vi "JSON text to Variant.vi"(6 "LVClass Serializer":refnum<class "JSONtext LVClass Serializer.lvclass">, 8 "error in (no error)":errorcluster, 9 "Data Type":variant, 10 "Offset":i32, 11 "JSON":string) -> (0 "error out":errorcluster, 1 "Variant out":variant)   [LabVIEW 2024, in "JSONtext.lvlib"]
doc: "Convert JSON to the LabVIEW Data Type entered.\n\nStrings or Arrays of strings marked with a leading \"<JSON>\" tag in their name (including inside clusters) are returnd as JSON. \n\nStrings or Arrays of strings marked with a leading \"<UTF8>\" tag in their name (including inside clusters) are returned encoded as UTF-8 (rather than the standard LabVIEW encoding)."
uses:
  JSONtext.lvlib
  JSONtext LVClass Serializer.lvclass
  Data Type.ctl
  Unescape JSON string.vi
  Get Number Text.vi
  NaN or null to Integer ERROR.vi
  Get JSON String.vi
  Base64 or Base64URL Decode.vi
  Get String.vi
  Advance past Line Ending.vi
  Advance past Number.vi
  Advance past String.vi
  Error Cluster From Error Code.vi
  NI_Data Type.lvlib
  JDP Utility.lvlib
  SetMap.lvlib
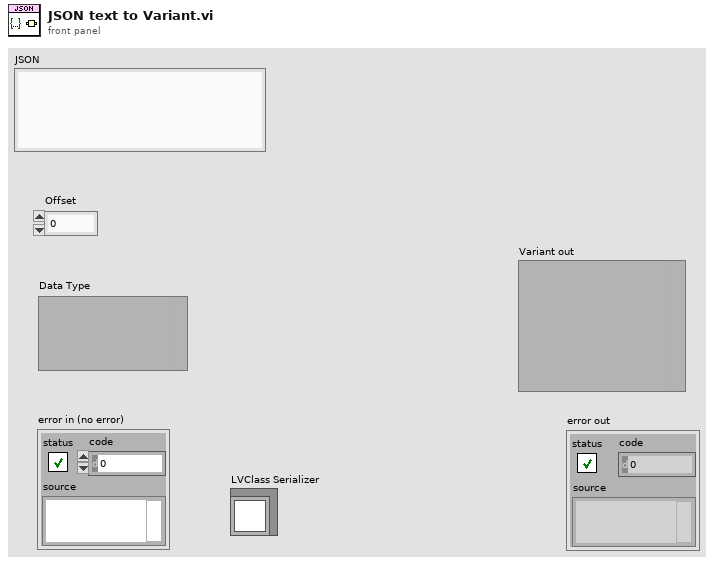
[diagram p1: front panel]
types:
  T1 = typedef "NI_Data Type.lvlib/Data Type.ctl" = enum8{"Invalid Type", "Void", "I8", "I16", "I32", "I64", "U8", "U16", "U32", "U64", "Single Float", "Double Float", "Extended Float", "Single Complex", "Double Complex", "Extended Complex", "Enum U8", "Enum U16", "Enum U32", "Enum U64", "Single Float With Unit", "Double Float With Unit", "Extended Float With Unit", "Single Complex with Unit", "Double Complex with Unit", "Extended Complex with Unit", "Boolean", "String", "Path", "Picture", "Tag", "Array", "Cluster", "Variant", "LV Variant", "Waveform", "Timestamp", "Digital Waveform", "Digital Data", "ExpressData", "Refnum", "External Data", "VI", "Poly VI", "LabVIEW Class Instance", "Fixed Point", "Set Collection", "Map Collection"}
  T2 = typedef "JSONtext.lvlib/Parsing State.ctl" = enum16{"Parser Error", "Object", "Array", "String", "Number/Other", "Leading Whitespace", "Object end", "Array end", "Value end"}
  T3 = typedef "JSONtext.lvlib/Tag Type.ctl" = enum16{"No Tag", "<JSON>", "<JOBJ>", "<UTF8>"}
  T4 = cluster{"Type":T1, "error out":errorcluster, "Tag":T3}[]
  T5 = typedef "JSONtext.lvlib/JSON Value Type.ctl" = enum16{"Not a JSON Value", "JSON Object", "JSON Array", "String", "Number", "true", "false", "null"}
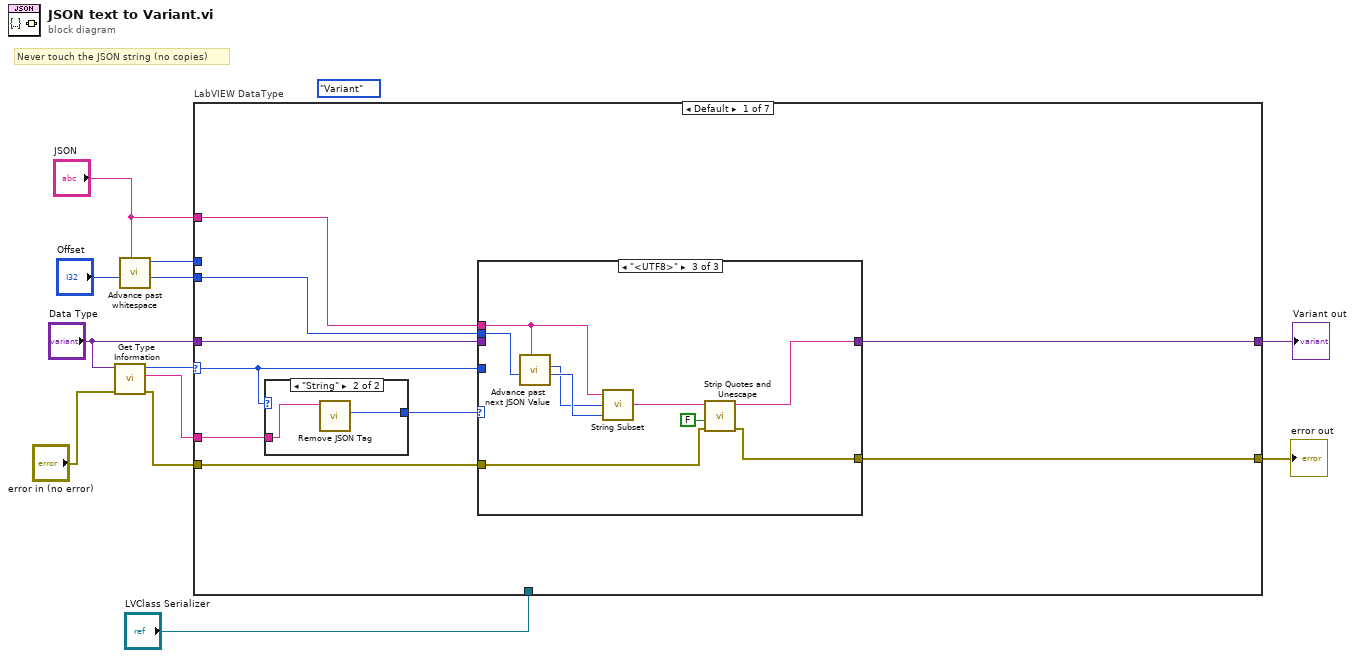
[diagram p0: block diagram]
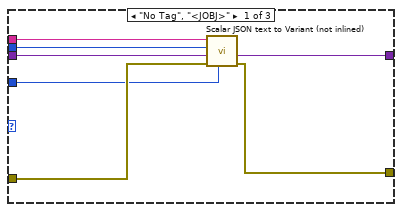
[diagram p2: hidden frame]
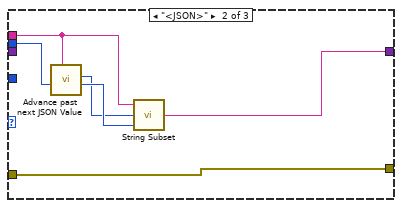
[diagram p3: hidden frame]
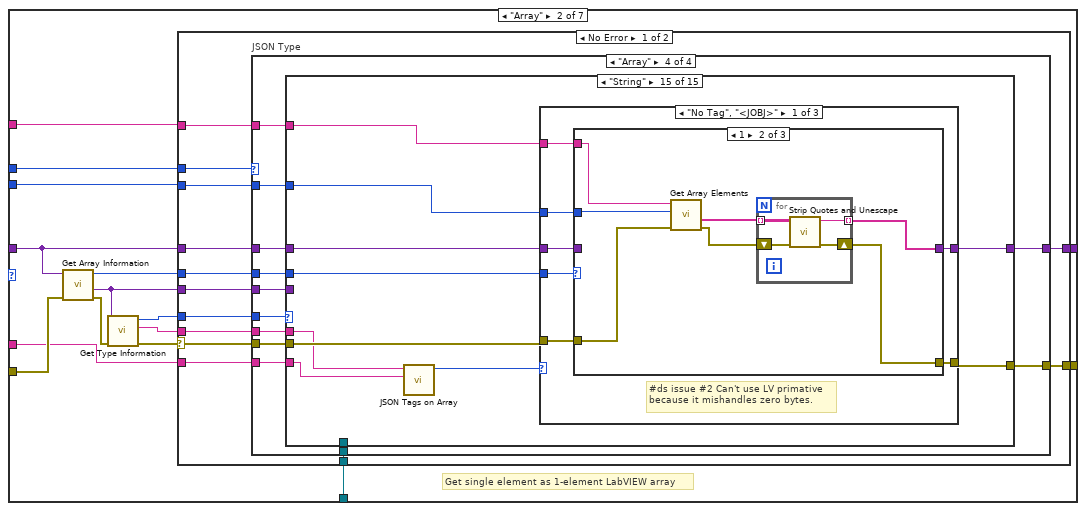
[diagram p5: hidden frame]
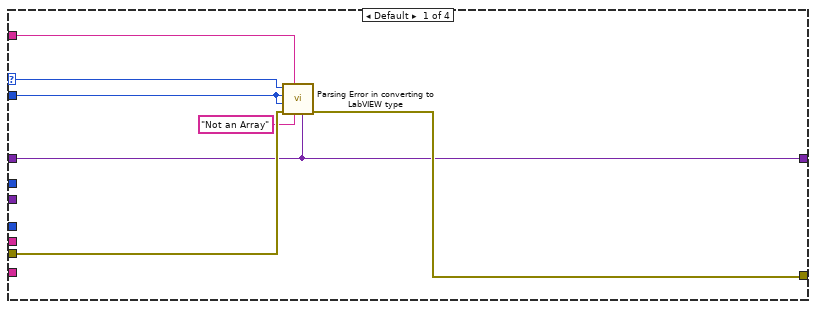
[diagram p6: hidden frame]
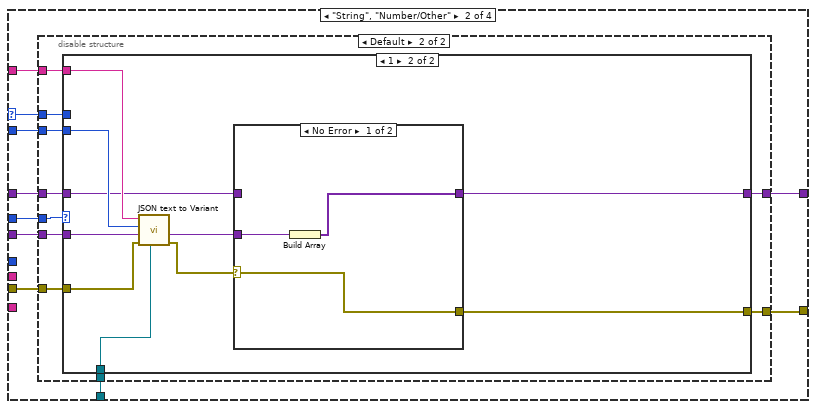
[diagram p7: hidden frame]
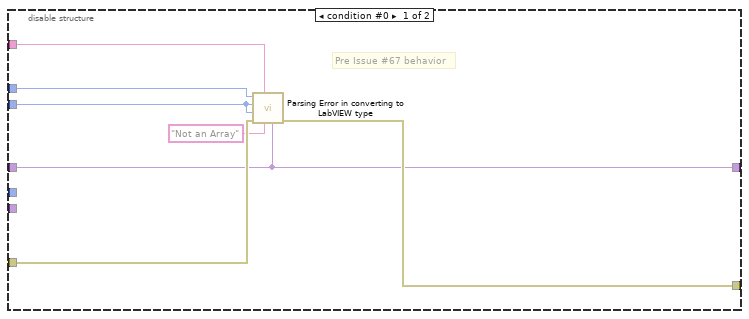
[diagram p8: hidden frame]
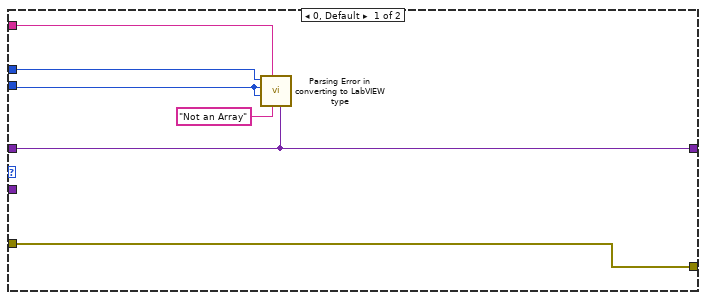
[diagram p9: hidden frame]
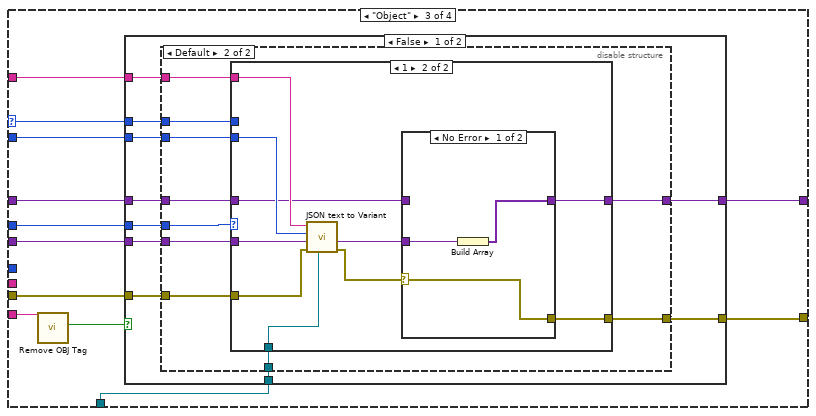
[diagram p11: hidden frame]
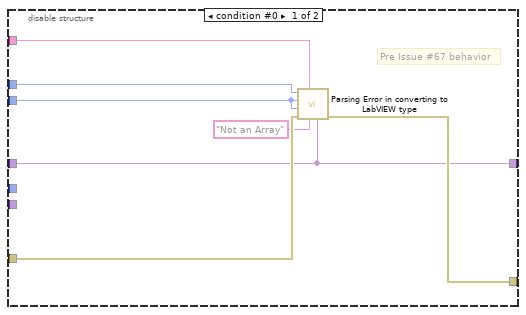
[diagram p12: hidden frame]
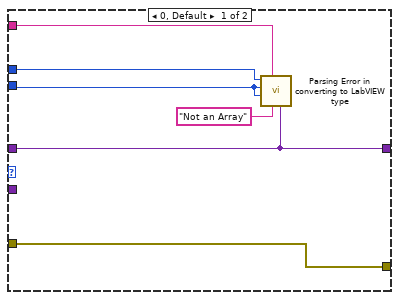
[diagram p13: hidden frame]
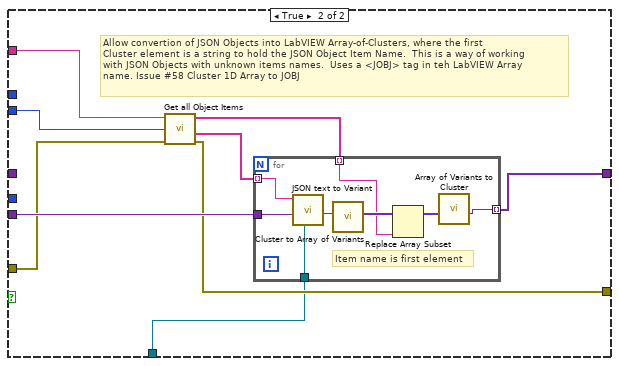
[diagram p15: hidden frame]
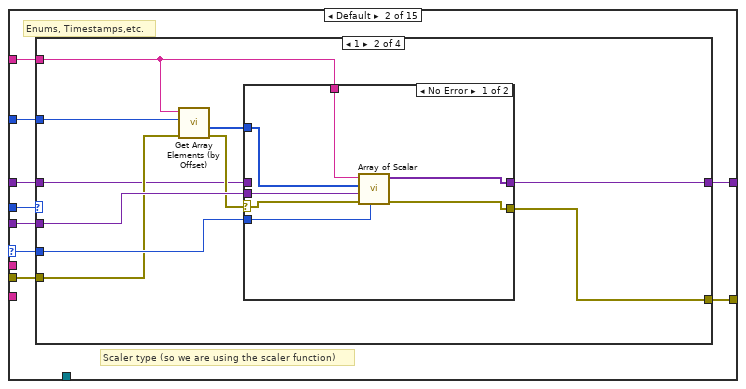
[diagram p17: hidden frame]
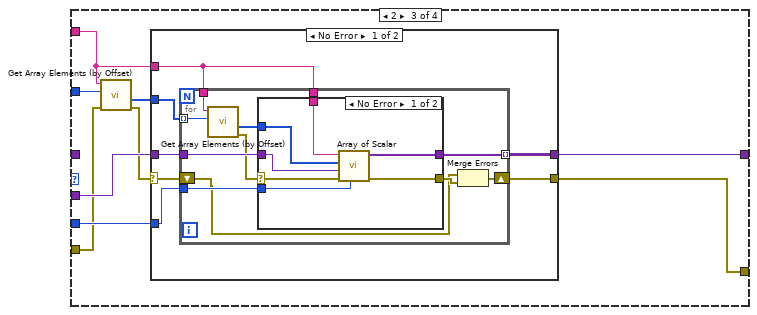
[diagram p20: hidden frame]
diagram:
  (unwired) Data_Type."Variant" ("Type")
  # "Never touch the JSON string (no copies)"
  n1 = call "Get Type Information.vi"("error in (no error)"="error in (no error)", "variant"="Data Type") -> ("error out"=w8:errorcluster, "name"=w2:string, "type"=w12:T1)  [unwired: 5 in, 2 out]
  n2 = call "Advance past whitespace.vi"("JSON"="JSON", "Offset"="Offset") -> ("Offset of first non-whitespace"=w5:i32, "Parser State"=w3:T2)  [unwired: 7 in, 1 out]
  n3 = case "LabVIEW DataType" shown="Default" w12 {
    selector: w12 -> [w14 _ _ _ _ _ w2257]
    tunnel: "Data Type" -> [w21 w53 w2187 w2195 w2226 w2237 w2259]
    tunnel: "JSON" -> [w19 w51 w2181 w2192 w2221 w2238 w2258]
    tunnel: [w16 w57 w2178 w2193 w2218 w2231 w2253] -> w9
    tunnel: w8 -> [w17 w60 w2186 w2194 w2225 w2235 w2254]
    tunnel: w5 -> [w18 w49 w2180 w2189 w2220 w2230 w2256]
    tunnel: [w20 w56 w2171 w2191 w2223 w2232 w2255] -> w7
    tunnel: w3 -> [_ w47 _ w2188 _ _ _]
    tunnel: w2 -> [w15 w50 _ _ _ _ _]
    tunnel: "LVClass Serializer" -> [_ w46 w2170 w2190 w2216 w2229 w2252]
    frame Default {
      n4 = case shown="\"String\"" w14 {
        tunnel: w15 -> [_ w45]
        tunnel: [_ w44] -> w13
        frame "Invalid Type", Default {
        }
        frame "String" {
          n5 = call "Remove JSON Tag.vi"("Name"=w45) -> ("Tag"=w44:T3)  [unwired: 9 in, 1 out]
        }
      }
      n6 = case shown="\"<UTF8>\"" w13 {
        tunnel: w21 -> [w28 _ _]
        tunnel: [w27 w30 w38] -> w20
        tunnel: w19 -> [w26 w31 w40]
        tunnel: w18 -> [w25 w34 w43]
        tunnel: w17 -> [w24 w29 w37]
        tunnel: [w23 w29 w36] -> w16
        tunnel: w14 -> [w22 _ _]
        frame "No Tag", "<JOBJ>" {
          n7 = call "Scalar JSON text to Variant (not inlined).vi"("Type"=w22, "error in (no error)"=w24, "Variant (Data Type)"=w28, "Offset (no whitespace)"=w25, "JSON"=w26) -> ("error out"=w23:errorcluster, "Variant out"=w27:variant)  [unwired: 5 in]
        }
        frame "<JSON>" {
          n8 = call "Advance past next JSON Value.vi"("JSON"=w31, "Offset"=w34) -> ("Offset out"=w33:i32, "Value start"=w32:i32)  [unwired: 7 in, 1 out]
          n9 = call "String Subset.vi"("Offset past End"=w33, "Start offset"=w32, "JSON"=w31) -> ("substring"=w30:string)  [unwired: 2 in]
        }
        frame "<UTF8>" {
          n10 = call "Advance past next JSON Value.vi"("JSON"=w40, "Offset"=w43) -> ("Offset out"=w42:i32, "Value start"=w41:i32)  [unwired: 7 in, 1 out]
          n11 = call "String Subset.vi"("Offset past End"=w42, "Start offset"=w41, "JSON"=w40) -> ("substring"=w39:string)  [unwired: 2 in]
          n12 = call "Strip Quotes and Unescape.vi"("error in (no error)"=w37, "To System Encoding (T)"=FALSE, "String"=w39) -> ("error out"=w36:errorcluster, "result string"=w38:string)  [unwired: 7 in]
        }
      }
    }
    frame "Array" {
      # "Get single element as 1-element LabVIEW array"
      n13 = call "Get Array Information.vi"("error in (no error)"=w60, "variant"=w53) -> ("error out"=w59:errorcluster, "array element data type"=w52:variant, "number of dimensions"=w54:i32)  [unwired: 6 in, 1 out]
      n14 = call "Get Type Information.vi"("error in (no error)"=w59, "variant"=w52) -> ("error out"=w58:errorcluster, "name"=w48:string, "type"=w55:T1)  [unwired: 5 in, 2 out]
      n15 = case shown="No Error" w58 {
        selector: w58 -> [w73 w2168]
        tunnel: [w72 w2168] -> w57
        tunnel: [w71 w2167] -> w56
        tunnel: w55 -> [w70 _]
        tunnel: w54 -> [w69 _]
        tunnel: w53 -> [w68 w2167]
        tunnel: w52 -> [w67 _]
        tunnel: w51 -> [w66 _]
        tunnel: w50 -> [w65 _]
        tunnel: w49 -> [w64 _]
        tunnel: w48 -> [w63 _]
        tunnel: w47 -> [w62 _]
        tunnel: w46 -> [w61 _]
        frame No Error {
          n16 = case "JSON Type" shown="\"Array\"" w62 {
            selector: w62 -> [w78 w88 w138 _]
            tunnel: w73 -> [w77 w87 w137 w217]
            tunnel: [w76 w86 w136 w216] -> w72
            tunnel: [w75 w83 w133 w215] -> w71
            tunnel: w70 -> [_ _ _ w214]
            tunnel: w69 -> [_ w82 w132 w213]
            tunnel: w68 -> [w75 w85 w135 w212]
            tunnel: w67 -> [_ w84 w134 w211]
            tunnel: w66 -> [w80 w90 w140 w210]
            tunnel: w65 -> [_ _ w130 w209]
            tunnel: w64 -> [w79 w89 w139 w208]
            tunnel: w63 -> [_ _ _ w207]
            tunnel: w61 -> [_ w81 w131 w206]
            frame Default {
              n17 = call "Parsing Error in converting to LabVIEW type.vi"("LV Type"=w75, "initial string"="Not an Array", "JSON"=w80, "error in (no error)"=w77, "Offset past match"=w79, "Value start"=w79, "State"=w78) -> ("error out"=w76:errorcluster)  [unwired: 4 in]
            }
            frame "String", "Number/Other" {
              n18 = disable-structure shown="Default" {
                disable-tunnel: w90 -> [w97 w106]
                disable-tunnel: w89 -> [w96 w105]
                disable-tunnel: w88 -> [w95 w99]
                disable-tunnel: w87 -> [w94 w104]
                disable-tunnel: [w93 w101] -> w86
                disable-tunnel: w85 -> [w91 w102]
                disable-tunnel: w84 -> [_ w107]
                disable-tunnel: [w91 w103] -> w83
                disable-tunnel: w82 -> [_ w100]
                disable-tunnel: w81 -> [_ w98]
                frame condition #0 {
                  # "Pre Issue #67 behavior"
                  n19 = call "Parsing Error in converting to LabVIEW type.vi"("LV Type"=w91, "initial string"="Not an Array", "JSON"=w97, "error in (no error)"=w94, "Offset past match"=w96, "Value start"=w96, "State"=w95) -> ("error out"=w93:errorcluster)  [unwired: 4 in]
                }
                frame condition #1 (active) {
                  n20 = case shown="1" w100 {
                    tunnel: w107 -> [_ w123]
                    tunnel: w106 -> [w112 w122]
                    tunnel: w105 -> [w110 w121]
                    tunnel: w104 -> [w108 w119]
                    tunnel: [w109 w117] -> w103
                    tunnel: w102 -> [w109 w116]
                    tunnel: [w108 w115] -> w101
                    tunnel: w99 -> [w111 _]
                    tunnel: w98 -> [_ w114]
                    frame 0, Default {
                      n21 = call "Parsing Error in converting to LabVIEW type.vi"("LV Type"=w109, "initial string"="Not an Array", "JSON"=w112, "Offset past match"=w110, "Value start"=w110, "State"=w111) -> ()  [unwired: 5 in, 1 out]
                    }
                    frame 1 {
                      n22 = call "JSON text to Variant.vi"("LVClass Serializer"=w114, "error in (no error)"=w119, "Data Type"=w123, "Offset"=w121, "JSON"=w122) -> ("error out"=w118:errorcluster, "Variant out"=w120:variant)  [unwired: 5 in]
                      n23 = case shown="No Error" w118 {
                        selector: w118 -> [w124 w127]
                        tunnel: w120 -> [w126 _]
                        tunnel: [w125 w128] -> w117
                        tunnel: w116 -> [_ w128]
                        tunnel: [w124 w127] -> w115
                        frame No Error {
                          n24 = Build Array(w126) -> (w125:variant[])
                        }
                        frame Error {
                        }
                      }
                    }
                  }
                }
              }
            }
            frame "Object" {
              n25 = call "Remove OBJ Tag.vi"("Name"=w130) -> ("tagged as Item Name in JSON Objects"=w129:bool)  [unwired: 9 in, 1 out]
              n26 = case shown="False" w129 {
                tunnel: w140 -> [w150 w195]
                tunnel: w139 -> [w149 w189]
                tunnel: w138 -> [w148 _]
                tunnel: w137 -> [w147 w196]
                tunnel: [w146 w193] -> w136
                tunnel: w135 -> [w145 _]
                tunnel: w134 -> [w144 w197]
                tunnel: [w143 w194] -> w133
                tunnel: w132 -> [w142 _]
                tunnel: w131 -> [w141 w192]
                frame False {
                  n27 = disable-structure shown="Default" {
                    disable-tunnel: w150 -> [w157 w166]
                    disable-tunnel: w149 -> [w156 w165]
                    disable-tunnel: w148 -> [w155 w159]
                    disable-tunnel: w147 -> [w154 w164]
                    disable-tunnel: [w153 w161] -> w146
                    disable-tunnel: w145 -> [w151 w162]
                    disable-tunnel: w144 -> [_ w167]
                    disable-tunnel: [w151 w163] -> w143
                    disable-tunnel: w142 -> [_ w160]
                    disable-tunnel: w141 -> [_ w158]
                    frame condition #0 {
                      # "Pre Issue #67 behavior"
                      n28 = call "Parsing Error in converting to LabVIEW type.vi"("LV Type"=w151, "initial string"="Not an Array", "JSON"=w157, "error in (no error)"=w154, "Offset past match"=w156, "Value start"=w156, "State"=w155) -> ("error out"=w153:errorcluster)  [unwired: 4 in]
                    }
                    frame condition #1 (active) {
                      n29 = case shown="1" w160 {
                        tunnel: w167 -> [_ w183]
                        tunnel: w166 -> [w172 w182]
                        tunnel: w165 -> [w170 w181]
                        tunnel: w164 -> [w168 w179]
                        tunnel: [w169 w177] -> w163
                        tunnel: w162 -> [w169 w176]
                        tunnel: [w168 w175] -> w161
                        tunnel: w159 -> [w171 _]
                        tunnel: w158 -> [_ w174]
                        frame 0, Default {
                          n30 = call "Parsing Error in converting to LabVIEW type.vi"("LV Type"=w169, "initial string"="Not an Array", "JSON"=w172, "Offset past match"=w170, "Value start"=w170, "State"=w171) -> ()  [unwired: 5 in, 1 out]
                        }
                        frame 1 {
                          n31 = call "JSON text to Variant.vi"("LVClass Serializer"=w174, "error in (no error)"=w179, "Data Type"=w183, "Offset"=w181, "JSON"=w182) -> ("error out"=w178:errorcluster, "Variant out"=w180:variant)  [unwired: 5 in]
                          n32 = case shown="No Error" w178 {
                            selector: w178 -> [w184 w187]
                            tunnel: w180 -> [w186 _]
                            tunnel: [w185 w188] -> w177
                            tunnel: w176 -> [_ w188]
                            tunnel: [w184 w187] -> w175
                            frame No Error {
                              n33 = Build Array(w186) -> (w185:variant[])
                            }
                            frame Error {
                            }
                          }
                        }
                      }
                    }
                  }
                }
                frame True {
                  # "Allow convertion of JSON Objects into LabVIEW Array-of-Clusters, where the first\nCluster element is a string to hold the JSON Object Item Name.  This is a way of working\nwith JSON Objects with unknown items names.  Uses a <JOBJ> tag in teh LabVIEW Array\nname. Issue #58 Cluster 1D Array to JOBJ"
                  n34 = call "Get all Object Items.vi"("error in (no error)"=w196, "Offset"=w189, "JSON"=w195) -> ("error out"=w193:errorcluster, "<JSON>"=w191:string[], "Item Names"=w190:string[])  [unwired: 5 in, 1 out]
                  n35 = for {
                    tunnel: w191 -> [w205] mode=indexing
                    tunnel: w197 -> [w204]
                    tunnel: w190 -> [w200] mode=indexing
                    tunnel: [w199] -> w194 mode=indexing
                    tunnel: w192 -> [w198]
                    # "Item name is first element"
                    n36 = call "JSON text to Variant.vi"("LVClass Serializer"=w198, "Data Type"=w204, "JSON"=w205) -> ("Variant out"=w202:variant)  [unwired: 7 in, 1 out]
                    n37 = call "Cluster to Array of Variants.vi"("Cluster"=w202) -> ("Array of Cluster Elements"=w201:variant[])  [unwired: 10 in]
                    n38 = Replace Array Subset(array=w201, new element=w200) -> (w203:variant[])  [unwired: 1 in]
                    n39 = call "Array of Variants to Cluster.vi"("Array of Variants"=w203) -> ("Cluster of Variants"=w199:variant)  [unwired: 10 in]
                  }
                }
              }
            }
            frame "Array" {
              n40 = case shown="\"String\"" w214 {
                selector: w214 -> [_ w220 w352 w491 w630 w769 w908 w1047 w1186 w1325 w1464 w1603 w1743 w1899 _]
                tunnel: w210 -> [_ w224 w356 w495 w634 w773 w912 w1051 w1190 w1329 w1468 w1607 w1747 w1903 w2062]
                tunnel: w217 -> [w218 w227 w359 w498 w637 w776 w915 w1054 w1193 w1332 w1471 w1610 w1750 w1906 w2061]
                tunnel: [w218 w228 w360 w499 w638 w777 w916 w1055 w1194 w1333 w1472 w1611 w1751 w1907 w2060] -> w216
                tunnel: [w219 w225 w357 w496 w635 w774 w913 w1052 w1191 w1330 w1469 w1608 w1748 w1904 w2059] -> w215
                tunnel: w213 -> [_ w223 w355 w494 w633 w772 w911 w1050 w1189 w1328 w1467 w1606 w1746 w1902 w2058]
                tunnel: w212 -> [w219 w222 w354 w493 w632 w771 w910 w1049 w1188 w1327 w1466 w1605 w1745 w1901 w2057]
                tunnel: w211 -> [_ w226 w358 w497 w636 w775 w914 w1053 w1192 w1331 w1470 w1609 w1749 w1905 _]
                tunnel: w208 -> [_ w221 w353 w492 w631 w770 w909 w1048 w1187 w1326 w1465 w1604 w1744 w1900 w2055]
                tunnel: w209 -> [_ _ _ _ _ _ _ _ _ _ _ _ _ _ w2056]
                tunnel: w207 -> [_ _ _ _ _ _ _ _ _ _ _ _ _ _ w2054]
                tunnel: w206 -> [_ _ _ _ _ _ _ _ _ _ _ _ w1742 w1898 _]
                frame "Invalid Type" {
                }
                frame Default {
                  # "Enums, Timestamps,etc."
                  # "Scaler type (so we are using the scaler function)"
                  n41 = case shown="1" w223 {
                    tunnel: [w229 w240 w254 w294] -> w228
                    tunnel: w227 -> [w229 w234 w252 w292]
                    tunnel: w226 -> [_ w239 w258 w298]
                    tunnel: [w230 w237 w256 w296] -> w225
                    tunnel: w221 -> [_ w236 w255 w295]
                    tunnel: w224 -> [_ w231 w250 w290]
                    tunnel: w222 -> [w230 w232 _ _]
                    tunnel: w220 -> [_ w235 w253 w293]
                    frame 0, Default {
                    }
                    frame 1 {
                      n42 = call "Get Array Elements (by Offset).vi"("error in (no error)"=w234, "Offset"=w236, "JSON"=w231) -> ("error out"=w233:errorcluster, "Element Offsets"=w238:i32[])  [unwired: 5 in, 2 out]
                      n43 = case shown="No Error" w233 {
                        selector: w233 -> [w243 w248]
                        tunnel: [w247 w248] -> w240
                        tunnel: w239 -> [w246 _]
                        tunnel: w238 -> [w245 _]
                        tunnel: [w244 w249] -> w237
                        tunnel: w235 -> [w241 _]
                        tunnel: w232 -> [_ w249]
                        tunnel: w231 -> [w242 _]
                        frame No Error {
                          n44 = call "Array of Scalar.vi"("Type"=w241, "error in (no error)"=w243, "Array Element Data Type"=w246, "Element Offsets"=w245, "JSON"=w242) -> ("error out"=w247:errorcluster, "Array"=w244:variant[])  [unwired: 5 in]
                        }
                        frame Error {
                        }
                      }
                    }
                    frame 2 {
                      n45 = call "Get Array Elements (by Offset).vi"("error in (no error)"=w252, "Offset"=w255, "JSON"=w250) -> ("error out"=w251:errorcluster, "Element Offsets"=w257:i32[])  [unwired: 5 in, 2 out]
                      n46 = case shown="No Error" w251 {
                        selector: w251 -> [w261 w289]
                        tunnel: w258 -> [w265 w288]
                        tunnel: w257 -> [w264 _]
                        tunnel: [w263 w288] -> w256
                        tunnel: [w259 w289] -> w254
                        tunnel: w253 -> [w262 _]
                        tunnel: w250 -> [w260 _]
                        frame No Error {
                          n47 = for {
                            tunnel: w265 -> [w275]
                            tunnel: w264 -> [w270] mode=indexing
                            tunnel: [w274] -> w263 mode=indexing
                            tunnel: w262 -> [w272]
                            tunnel: w260 -> [w269]
                            tunnel: w260 -> [w268]
                            shift-right: [w267] -> w259
                            shift-left: w261 -> [w266]
                            n48 = call "Get Array Elements (by Offset).vi"("Offset"=w270, "JSON"=w269) -> ("error out"=w271:errorcluster, "Element Offsets"=w273:i32[])  [unwired: 6 in, 2 out]
                            n49 = case shown="No Error" w271 {
                              selector: w271 -> [w279 w287]
                              tunnel: [w280 w287] -> w276
                              tunnel: w275 -> [w278 w285]
                              tunnel: [w281 w284] -> w274
                              tunnel: w273 -> [w282 _]
                              tunnel: w272 -> [w277 _]
                              tunnel: w268 -> [w283 _]
                              frame No Error {
                                n50 = call "Array of Scalar.vi"("Type"=w277, "error in (no error)"=w279, "Array Element Data Type"=w278, "Element Offsets"=w282, "JSON"=w283) -> ("error out"=w280:errorcluster, "Array"=w281:variant[])  [unwired: 5 in]
                              }
                              frame Error {
                                n51 = Initialize Array(w285, 0 ("dimension size")) -> (w284:variant[])
                              }
                            }
                            n52 = Merge Errors(w266, w276) -> (w267:errorcluster)
                          }
                        }
                        frame Error {
                        }
                      }
                    }
                    frame 3 {
                      n53 = call "Get Array Elements (by Offset).vi"("error in (no error)"=w292, "Offset"=w295, "JSON"=w290) -> ("error out"=w291:errorcluster, "Element Offsets"=w297:i32[])  [unwired: 5 in, 2 out]
                      n54 = case shown="No Error" w291 {
                        selector: w291 -> [w301 w351]
                        tunnel: w298 -> [w305 w350]
                        tunnel: w297 -> [w304 _]
                        tunnel: [w303 w350] -> w296
                        tunnel: [w299 w351] -> w294
                        tunnel: w293 -> [w302 _]
                        tunnel: w290 -> [w300 _]
                        frame No Error {
                          n55 = for {
                            tunnel: w305 -> [w315]
                            tunnel: w304 -> [w310] mode=indexing
                            tunnel: [w314] -> w303 mode=indexing
                            tunnel: w302 -> [w312]
                            tunnel: w300 -> [w309]
                            tunnel: w300 -> [w308]
                            shift-right: [w307] -> w299
                            shift-left: w301 -> [w306]
                            n56 = call "Get Array Elements (by Offset).vi"("Offset"=w310, "JSON"=w309) -> ("error out"=w311:errorcluster, "Element Offsets"=w313:i32[])  [unwired: 6 in, 2 out]
                            n57 = case shown="No Error" w311 {
                              selector: w311 -> [w317 w349]
                              tunnel: [w319 w349] -> w316
                              tunnel: w315 -> [w323 w348]
                              tunnel: [w318 w346] -> w314
                              tunnel: w313 -> [w322 _]
                              tunnel: w312 -> [w320 _]
                              tunnel: w308 -> [w321 _]
                              frame No Error {
                                n58 = for {
                                tunnel: w323 -> [w333]
                                tunnel: w322 -> [w328] mode=indexing
                                tunnel: [w332] -> w318 mode=indexing
                                tunnel: w320 -> [w330]
                                tunnel: w321 -> [w327]
                                tunnel: w321 -> [w326]
                                shift-right: [w325] -> w319
                                shift-left: w317 -> [w324]
                                n59 = call "Get Array Elements (by Offset).vi"("Offset"=w328, "JSON"=w327) -> ("error out"=w329:errorcluster, "Element Offsets"=w331:i32[])  [unwired: 6 in, 2 out]
                                n60 = case shown="No Error" w329 {
                                selector: w329 -> [w339 w345]
                                tunnel: [w340 w345] -> w334
                                tunnel: w333 -> [w338 w344]
                                tunnel: [w341 w342] -> w332
                                tunnel: w331 -> [w337 _]
                                tunnel: w330 -> [w335 _]
                                tunnel: w326 -> [w336 _]
                                frame No Error {
                                n61 = call "Array of Scalar.vi"("Type"=w335, "error in (no error)"=w339, "Array Element Data Type"=w338, "Element Offsets"=w337, "JSON"=w336) -> ("error out"=w340:errorcluster, "Array"=w341:variant[])  [unwired: 5 in]
                                }
                                frame Error {
                                n62 = Initialize Array(w344, 0 ("dimension size")) -> (w342:variant[])
                                }
                                }
                                n63 = Merge Errors(w324, w334) -> (w325:errorcluster)
                                }
                              }
                              frame Error {
                                w347 = 0 ("dimension size")
                                n64 = Initialize Array(w348, w347, w347) -> (w346:variant[][])
                              }
                            }
                            n65 = Merge Errors(w306, w316) -> (w307:errorcluster)
                          }
                        }
                        frame Error {
                        }
                      }
                    }
                  }
                }
                frame "Double Float", "Extended Float", "Double Float With Unit", "Extended Float With Unit" {
                  # "Scaler type (so we are using the inlined function)"
                  n66 = case shown="3" w355 {
                    tunnel: [w361 w372 w391 w433] -> w360
                    tunnel: w359 -> [w361 w366 w389 w431]
                    tunnel: w358 -> [_ w371 w395 w437]
                    tunnel: [w362 w369 w393 w435] -> w357
                    tunnel: w353 -> [_ w368 w392 w434]
                    tunnel: w356 -> [_ w363 w387 w429]
                    tunnel: w354 -> [w362 w364 _ _]
                    tunnel: w352 -> [_ w367 w390 w432]
                    frame 0, Default {
                    }
                    frame 1 {
                      n67 = call "Get Array Elements (by Offset).vi"("error in (no error)"=w366, "Offset"=w368, "JSON"=w363) -> ("error out"=w365:errorcluster, "Element Offsets"=w370:i32[])  [unwired: 5 in, 2 out]
                      n68 = case shown="No Error" w365 {
                        selector: w365 -> [w374 w386]
                        tunnel: [w379 w386] -> w372
                        tunnel: w371 -> [w378 _]
                        tunnel: w370 -> [w377 _]
                        tunnel: [w376 _] -> w369
                        tunnel: w367 -> [w375 _]
                        tunnel: w364 -> [_ _]
                        tunnel: w363 -> [w373 _]
                        frame No Error {
                          n69 = for {
                            tunnel: w378 -> [_]
                            tunnel: [w381] -> w376 mode=indexing
                            tunnel: w377 -> [w382] mode=indexing
                            tunnel: w375 -> [_]
                            tunnel: w373 -> [w383]
                            shift-right: [w385] -> w379
                            shift-left: w374 -> [w384]
                            n70 = call "Get DBL.vi"("Offset"=w382, "JSON"=w383) -> ("error out"=w380:errorcluster, "Number"=w381:dbl)  [unwired: 7 in, 1 out]
                            n71 = Merge Errors(w384, w380) -> (w385:errorcluster)
                          }
                        }
                        frame Error {
                        }
                      }
                    }
                    frame 2 {
                      n72 = call "Get Array Elements (by Offset).vi"("error in (no error)"=w389, "Offset"=w392, "JSON"=w387) -> ("error out"=w388:errorcluster, "Element Offsets"=w394:i32[])  [unwired: 5 in, 2 out]
                      n73 = case shown="No Error" w388 {
                        selector: w388 -> [w398 w428]
                        tunnel: w395 -> [w402 _]
                        tunnel: w394 -> [w401 _]
                        tunnel: [w400 _] -> w393
                        tunnel: [w396 w428] -> w391
                        tunnel: w390 -> [w399 _]
                        tunnel: w387 -> [w397 _]
                        frame No Error {
                          n74 = for {
                            tunnel: w402 -> [w412]
                            tunnel: w401 -> [w407] mode=indexing
                            tunnel: [w411] -> w400 mode=indexing
                            tunnel: w399 -> [w409]
                            tunnel: w397 -> [w406]
                            tunnel: w397 -> [w405]
                            shift-right: [w404] -> w396
                            shift-left: w398 -> [w403]
                            n75 = call "Get Array Elements (by Offset).vi"("Offset"=w407, "JSON"=w406) -> ("error out"=w408:errorcluster, "Element Offsets"=w410:i32[])  [unwired: 6 in, 2 out]
                            n76 = case shown="No Error" w408 {
                              selector: w408 -> [w416 w427]
                              tunnel: [w414 w427] -> w413
                              tunnel: w412 -> [w420 _]
                              tunnel: [w419 _] -> w411
                              tunnel: w410 -> [w418 _]
                              tunnel: w409 -> [w417 _]
                              tunnel: w405 -> [w415 _]
                              frame No Error {
                                n77 = for {
                                tunnel: w420 -> [_]
                                tunnel: [w421] -> w419 mode=indexing
                                tunnel: w418 -> [w423] mode=indexing
                                tunnel: w417 -> [_]
                                tunnel: w415 -> [w424]
                                shift-right: [w426] -> w414
                                shift-left: w416 -> [w425]
                                n78 = call "Get DBL.vi"("Offset"=w423, "JSON"=w424) -> ("error out"=w422:errorcluster, "Number"=w421:dbl)  [unwired: 7 in, 1 out]
                                n79 = Merge Errors(w425, w422) -> (w426:errorcluster)
                                }
                              }
                              frame Error {
                              }
                            }
                            n80 = Merge Errors(w403, w413) -> (w404:errorcluster)
                          }
                        }
                        frame Error {
                        }
                      }
                    }
                    frame 3 {
                      n81 = call "Get Array Elements (by Offset).vi"("error in (no error)"=w431, "Offset"=w434, "JSON"=w429) -> ("error out"=w430:errorcluster, "Element Offsets"=w436:i32[])  [unwired: 5 in, 2 out]
                      n82 = case shown="No Error" w430 {
                        selector: w430 -> [w440 w490]
                        tunnel: w437 -> [w444 w489]
                        tunnel: w436 -> [w443 _]
                        tunnel: [w442 w489] -> w435
                        tunnel: [w438 w490] -> w433
                        tunnel: w432 -> [w441 _]
                        tunnel: w429 -> [w439 _]
                        frame No Error {
                          n83 = for {
                            tunnel: w444 -> [w454]
                            tunnel: w443 -> [w449] mode=indexing
                            tunnel: [w453] -> w442 mode=indexing
                            tunnel: w441 -> [w451]
                            tunnel: w439 -> [w448]
                            tunnel: w439 -> [w447]
                            shift-right: [w446] -> w438
                            shift-left: w440 -> [w445]
                            n84 = call "Get Array Elements (by Offset).vi"("Offset"=w449, "JSON"=w448) -> ("error out"=w450:errorcluster, "Element Offsets"=w452:i32[])  [unwired: 6 in, 2 out]
                            n85 = case shown="No Error" w450 {
                              selector: w450 -> [w456 w488]
                              tunnel: [w458 w488] -> w455
                              tunnel: w454 -> [w462 _]
                              tunnel: [w457 _] -> w453
                              tunnel: w452 -> [w461 _]
                              tunnel: w451 -> [w459 _]
                              tunnel: w447 -> [w460 _]
                              frame No Error {
                                n86 = for {
                                tunnel: w462 -> [w472]
                                tunnel: w461 -> [w467] mode=indexing
                                tunnel: [w471] -> w457 mode=indexing
                                tunnel: w459 -> [w469]
                                tunnel: w460 -> [w466]
                                tunnel: w460 -> [w465]
                                shift-right: [w464] -> w458
                                shift-left: w456 -> [w463]
                                n87 = call "Get Array Elements (by Offset).vi"("Offset"=w467, "JSON"=w466) -> ("error out"=w468:errorcluster, "Element Offsets"=w470:i32[])  [unwired: 6 in, 2 out]
                                n88 = case shown="No Error" w468 {
                                selector: w468 -> [w476 w487]
                                tunnel: [w474 w487] -> w473
                                tunnel: w472 -> [w480 _]
                                tunnel: [w479 _] -> w471
                                tunnel: w470 -> [w478 _]
                                tunnel: w469 -> [w477 _]
                                tunnel: w465 -> [w475 _]
                                frame No Error {
                                n89 = for {
                                tunnel: w480 -> [_]
                                tunnel: [w481] -> w479 mode=indexing
                                tunnel: w478 -> [w484] mode=indexing
                                tunnel: w477 -> [_]
                                tunnel: w475 -> [w485]
                                shift-right: [w486] -> w474
                                shift-left: w476 -> [w483]
                                n90 = call "Get DBL.vi"("Offset"=w484, "JSON"=w485) -> ("error out"=w482:errorcluster, "Number"=w481:dbl)  [unwired: 7 in, 1 out]
                                n91 = Merge Errors(w483, w482) -> (w486:errorcluster)
                                }
                                }
                                frame Error {
                                }
                                }
                                n92 = Merge Errors(w463, w473) -> (w464:errorcluster)
                                }
                              }
                              frame Error {
                              }
                            }
                            n93 = Merge Errors(w445, w455) -> (w446:errorcluster)
                          }
                        }
                        frame Error {
                        }
                      }
                    }
                  }
                }
                frame "Single Float", "Single Float With Unit" {
                  # "Scaler type (so we are using the inlined function)"
                  n94 = case shown="3" w494 {
                    tunnel: [w500 w511 w530 w572] -> w499
                    tunnel: w498 -> [w500 w505 w528 w570]
                    tunnel: w497 -> [_ w510 w534 w576]
                    tunnel: [w501 w508 w532 w574] -> w496
                    tunnel: w492 -> [_ w507 w531 w573]
                    tunnel: w495 -> [_ w502 w526 w568]
                    tunnel: w493 -> [w501 w503 _ _]
                    tunnel: w491 -> [_ w506 w529 w571]
                    frame 0, Default {
                    }
                    frame 1 {
                      n95 = call "Get Array Elements (by Offset).vi"("error in (no error)"=w505, "Offset"=w507, "JSON"=w502) -> ("error out"=w504:errorcluster, "Element Offsets"=w509:i32[])  [unwired: 5 in, 2 out]
                      n96 = case shown="No Error" w504 {
                        selector: w504 -> [w513 w525]
                        tunnel: [w518 w525] -> w511
                        tunnel: w510 -> [w517 _]
                        tunnel: w509 -> [w516 _]
                        tunnel: [w515 _] -> w508
                        tunnel: w506 -> [w514 _]
                        tunnel: w503 -> [_ _]
                        tunnel: w502 -> [w512 _]
                        frame No Error {
                          n97 = for {
                            tunnel: w517 -> [_]
                            tunnel: [w520] -> w515 mode=indexing
                            tunnel: w516 -> [w521] mode=indexing
                            tunnel: w514 -> [_]
                            tunnel: w512 -> [w522]
                            shift-right: [w524] -> w518
                            shift-left: w513 -> [w523]
                            n98 = call "Get SGL.vi"("Offset"=w521, "JSON"=w522) -> ("error out"=w519:errorcluster, "Number"=w520:sgl)  [unwired: 7 in, 1 out]
                            n99 = Merge Errors(w523, w519) -> (w524:errorcluster)
                          }
                        }
                        frame Error {
                        }
                      }
                    }
                    frame 2 {
                      n100 = call "Get Array Elements (by Offset).vi"("error in (no error)"=w528, "Offset"=w531, "JSON"=w526) -> ("error out"=w527:errorcluster, "Element Offsets"=w533:i32[])  [unwired: 5 in, 2 out]
                      n101 = case shown="No Error" w527 {
                        selector: w527 -> [w537 w567]
                        tunnel: w534 -> [w541 _]
                        tunnel: w533 -> [w540 _]
                        tunnel: [w539 _] -> w532
                        tunnel: [w535 w567] -> w530
                        tunnel: w529 -> [w538 _]
                        tunnel: w526 -> [w536 _]
                        frame No Error {
                          n102 = for {
                            tunnel: w541 -> [w551]
                            tunnel: w540 -> [w546] mode=indexing
                            tunnel: [w550] -> w539 mode=indexing
                            tunnel: w538 -> [w548]
                            tunnel: w536 -> [w545]
                            tunnel: w536 -> [w544]
                            shift-right: [w543] -> w535
                            shift-left: w537 -> [w542]
                            n103 = call "Get Array Elements (by Offset).vi"("Offset"=w546, "JSON"=w545) -> ("error out"=w547:errorcluster, "Element Offsets"=w549:i32[])  [unwired: 6 in, 2 out]
                            n104 = case shown="No Error" w547 {
                              selector: w547 -> [w555 w566]
                              tunnel: [w553 w566] -> w552
                              tunnel: w551 -> [w559 _]
                              tunnel: [w558 _] -> w550
                              tunnel: w549 -> [w557 _]
                              tunnel: w548 -> [w556 _]
                              tunnel: w544 -> [w554 _]
                              frame No Error {
                                n105 = for {
                                tunnel: w559 -> [_]
                                tunnel: [w560] -> w558 mode=indexing
                                tunnel: w557 -> [w562] mode=indexing
                                tunnel: w556 -> [_]
                                tunnel: w554 -> [w563]
                                shift-right: [w565] -> w553
                                shift-left: w555 -> [w564]
                                n106 = call "Get SGL.vi"("Offset"=w562, "JSON"=w563) -> ("error out"=w561:errorcluster, "Number"=w560:sgl)  [unwired: 7 in, 1 out]
                                n107 = Merge Errors(w564, w561) -> (w565:errorcluster)
                                }
                              }
                              frame Error {
                              }
                            }
                            n108 = Merge Errors(w542, w552) -> (w543:errorcluster)
                          }
                        }
                        frame Error {
                        }
                      }
                    }
                    frame 3 {
                      n109 = call "Get Array Elements (by Offset).vi"("error in (no error)"=w570, "Offset"=w573, "JSON"=w568) -> ("error out"=w569:errorcluster, "Element Offsets"=w575:i32[])  [unwired: 5 in, 2 out]
                      n110 = case shown="No Error" w569 {
                        selector: w569 -> [w579 w629]
                        tunnel: w576 -> [w583 w628]
                        tunnel: w575 -> [w582 _]
                        tunnel: [w581 w628] -> w574
                        tunnel: [w577 w629] -> w572
                        tunnel: w571 -> [w580 _]
                        tunnel: w568 -> [w578 _]
                        frame No Error {
                          n111 = for {
                            tunnel: w583 -> [w593]
                            tunnel: w582 -> [w588] mode=indexing
                            tunnel: [w592] -> w581 mode=indexing
                            tunnel: w580 -> [w590]
                            tunnel: w578 -> [w587]
                            tunnel: w578 -> [w586]
                            shift-right: [w585] -> w577
                            shift-left: w579 -> [w584]
                            n112 = call "Get Array Elements (by Offset).vi"("Offset"=w588, "JSON"=w587) -> ("error out"=w589:errorcluster, "Element Offsets"=w591:i32[])  [unwired: 6 in, 2 out]
                            n113 = case shown="No Error" w589 {
                              selector: w589 -> [w595 w627]
                              tunnel: [w597 w627] -> w594
                              tunnel: w593 -> [w601 _]
                              tunnel: [w596 _] -> w592
                              tunnel: w591 -> [w600 _]
                              tunnel: w590 -> [w598 _]
                              tunnel: w586 -> [w599 _]
                              frame No Error {
                                n114 = for {
                                tunnel: w601 -> [w611]
                                tunnel: w600 -> [w606] mode=indexing
                                tunnel: [w610] -> w596 mode=indexing
                                tunnel: w598 -> [w608]
                                tunnel: w599 -> [w605]
                                tunnel: w599 -> [w604]
                                shift-right: [w603] -> w597
                                shift-left: w595 -> [w602]
                                n115 = call "Get Array Elements (by Offset).vi"("Offset"=w606, "JSON"=w605) -> ("error out"=w607:errorcluster, "Element Offsets"=w609:i32[])  [unwired: 6 in, 2 out]
                                n116 = case shown="No Error" w607 {
                                selector: w607 -> [w615 w626]
                                tunnel: [w613 w626] -> w612
                                tunnel: w611 -> [w619 _]
                                tunnel: [w618 _] -> w610
                                tunnel: w609 -> [w617 _]
                                tunnel: w608 -> [w616 _]
                                tunnel: w604 -> [w614 _]
                                frame No Error {
                                n117 = for {
                                tunnel: w619 -> [_]
                                tunnel: [w620] -> w618 mode=indexing
                                tunnel: w617 -> [w623] mode=indexing
                                tunnel: w616 -> [_]
                                tunnel: w614 -> [w624]
                                shift-right: [w625] -> w613
                                shift-left: w615 -> [w622]
                                n118 = call "Get SGL.vi"("Offset"=w623, "JSON"=w624) -> ("error out"=w621:errorcluster, "Number"=w620:sgl)  [unwired: 7 in, 1 out]
                                n119 = Merge Errors(w622, w621) -> (w625:errorcluster)
                                }
                                }
                                frame Error {
                                }
                                }
                                n120 = Merge Errors(w602, w612) -> (w603:errorcluster)
                                }
                              }
                              frame Error {
                              }
                            }
                            n121 = Merge Errors(w584, w594) -> (w585:errorcluster)
                          }
                        }
                        frame Error {
                        }
                      }
                    }
                  }
                }
                frame "I8" {
                  n122 = case shown="3" w633 {
                    tunnel: [w639 w650 w669 w711] -> w638
                    tunnel: w637 -> [w639 w644 w667 w709]
                    tunnel: w636 -> [_ w649 w673 w715]
                    tunnel: [w640 w647 w671 w713] -> w635
                    tunnel: w631 -> [_ w646 w670 w712]
                    tunnel: w634 -> [_ w641 w665 w707]
                    tunnel: w632 -> [w640 w642 _ _]
                    tunnel: w630 -> [_ w645 w668 w710]
                    frame 0, Default {
                    }
                    frame 1 {
                      n123 = call "Get Array Elements (by Offset).vi"("error in (no error)"=w644, "Offset"=w646, "JSON"=w641) -> ("error out"=w643:errorcluster, "Element Offsets"=w648:i32[])  [unwired: 5 in, 2 out]
                      n124 = case shown="No Error" w643 {
                        selector: w643 -> [w652 w664]
                        tunnel: [w657 w664] -> w650
                        tunnel: w649 -> [w656 _]
                        tunnel: w648 -> [w655 _]
                        tunnel: [w654 _] -> w647
                        tunnel: w645 -> [w653 _]
                        tunnel: w642 -> [_ _]
                        tunnel: w641 -> [w651 _]
                        frame No Error {
                          n125 = for {
                            tunnel: w656 -> [_]
                            tunnel: [w659] -> w654 mode=indexing
                            tunnel: w655 -> [w660] mode=indexing
                            tunnel: w653 -> [_]
                            tunnel: w651 -> [w661]
                            shift-right: [w663] -> w657
                            shift-left: w652 -> [w662]
                            n126 = call "Get I8.vi"("Offset"=w660, "JSON"=w661) -> ("error out"=w658:errorcluster, "Number"=w659:i8)  [unwired: 7 in, 1 out]
                            n127 = Merge Errors(w662, w658) -> (w663:errorcluster)
                          }
                        }
                        frame Error {
                        }
                      }
                    }
                    frame 2 {
                      n128 = call "Get Array Elements (by Offset).vi"("error in (no error)"=w667, "Offset"=w670, "JSON"=w665) -> ("error out"=w666:errorcluster, "Element Offsets"=w672:i32[])  [unwired: 5 in, 2 out]
                      n129 = case shown="No Error" w666 {
                        selector: w666 -> [w676 w706]
                        tunnel: w673 -> [w680 _]
                        tunnel: w672 -> [w679 _]
                        tunnel: [w678 _] -> w671
                        tunnel: [w674 w706] -> w669
                        tunnel: w668 -> [w677 _]
                        tunnel: w665 -> [w675 _]
                        frame No Error {
                          n130 = for {
                            tunnel: w680 -> [w690]
                            tunnel: w679 -> [w685] mode=indexing
                            tunnel: [w689] -> w678 mode=indexing
                            tunnel: w677 -> [w687]
                            tunnel: w675 -> [w684]
                            tunnel: w675 -> [w683]
                            shift-right: [w682] -> w674
                            shift-left: w676 -> [w681]
                            n131 = call "Get Array Elements (by Offset).vi"("Offset"=w685, "JSON"=w684) -> ("error out"=w686:errorcluster, "Element Offsets"=w688:i32[])  [unwired: 6 in, 2 out]
                            n132 = case shown="No Error" w686 {
                              selector: w686 -> [w694 w705]
                              tunnel: [w692 w705] -> w691
                              tunnel: w690 -> [w698 _]
                              tunnel: [w697 _] -> w689
                              tunnel: w688 -> [w696 _]
                              tunnel: w687 -> [w695 _]
                              tunnel: w683 -> [w693 _]
                              frame No Error {
                                n133 = for {
                                tunnel: w698 -> [_]
                                tunnel: [w699] -> w697 mode=indexing
                                tunnel: w696 -> [w701] mode=indexing
                                tunnel: w695 -> [_]
                                tunnel: w693 -> [w702]
                                shift-right: [w704] -> w692
                                shift-left: w694 -> [w703]
                                n134 = call "Get I8.vi"("Offset"=w701, "JSON"=w702) -> ("error out"=w700:errorcluster, "Number"=w699:i8)  [unwired: 7 in, 1 out]
                                n135 = Merge Errors(w703, w700) -> (w704:errorcluster)
                                }
                              }
                              frame Error {
                              }
                            }
                            n136 = Merge Errors(w681, w691) -> (w682:errorcluster)
                          }
                        }
                        frame Error {
                        }
                      }
                    }
                    frame 3 {
                      n137 = call "Get Array Elements (by Offset).vi"("error in (no error)"=w709, "Offset"=w712, "JSON"=w707) -> ("error out"=w708:errorcluster, "Element Offsets"=w714:i32[])  [unwired: 5 in, 2 out]
                      n138 = case shown="No Error" w708 {
                        selector: w708 -> [w718 w768]
                        tunnel: w715 -> [w722 w767]
                        tunnel: w714 -> [w721 _]
                        tunnel: [w720 w767] -> w713
                        tunnel: [w716 w768] -> w711
                        tunnel: w710 -> [w719 _]
                        tunnel: w707 -> [w717 _]
                        frame No Error {
                          n139 = for {
                            tunnel: w722 -> [w732]
                            tunnel: w721 -> [w727] mode=indexing
                            tunnel: [w731] -> w720 mode=indexing
                            tunnel: w719 -> [w729]
                            tunnel: w717 -> [w726]
                            tunnel: w717 -> [w725]
                            shift-right: [w724] -> w716
                            shift-left: w718 -> [w723]
                            n140 = call "Get Array Elements (by Offset).vi"("Offset"=w727, "JSON"=w726) -> ("error out"=w728:errorcluster, "Element Offsets"=w730:i32[])  [unwired: 6 in, 2 out]
                            n141 = case shown="No Error" w728 {
                              selector: w728 -> [w734 w766]
                              tunnel: [w736 w766] -> w733
                              tunnel: w732 -> [w740 _]
                              tunnel: [w735 _] -> w731
                              tunnel: w730 -> [w739 _]
                              tunnel: w729 -> [w737 _]
                              tunnel: w725 -> [w738 _]
                              frame No Error {
                                n142 = for {
                                tunnel: w740 -> [w750]
                                tunnel: w739 -> [w745] mode=indexing
                                tunnel: [w749] -> w735 mode=indexing
                                tunnel: w737 -> [w747]
                                tunnel: w738 -> [w744]
                                tunnel: w738 -> [w743]
                                shift-right: [w742] -> w736
                                shift-left: w734 -> [w741]
                                n143 = call "Get Array Elements (by Offset).vi"("Offset"=w745, "JSON"=w744) -> ("error out"=w746:errorcluster, "Element Offsets"=w748:i32[])  [unwired: 6 in, 2 out]
                                n144 = case shown="No Error" w746 {
                                selector: w746 -> [w754 w765]
                                tunnel: [w752 w765] -> w751
                                tunnel: w750 -> [w758 _]
                                tunnel: [w757 _] -> w749
                                tunnel: w748 -> [w756 _]
                                tunnel: w747 -> [w755 _]
                                tunnel: w743 -> [w753 _]
                                frame No Error {
                                n145 = for {
                                tunnel: w758 -> [_]
                                tunnel: [w759] -> w757 mode=indexing
                                tunnel: w756 -> [w762] mode=indexing
                                tunnel: w755 -> [_]
                                tunnel: w753 -> [w763]
                                shift-right: [w764] -> w752
                                shift-left: w754 -> [w761]
                                n146 = call "Get I8.vi"("Offset"=w762, "JSON"=w763) -> ("error out"=w760:errorcluster, "Number"=w759:i8)  [unwired: 7 in, 1 out]
                                n147 = Merge Errors(w761, w760) -> (w764:errorcluster)
                                }
                                }
                                frame Error {
                                }
                                }
                                n148 = Merge Errors(w741, w751) -> (w742:errorcluster)
                                }
                              }
                              frame Error {
                              }
                            }
                            n149 = Merge Errors(w723, w733) -> (w724:errorcluster)
                          }
                        }
                        frame Error {
                        }
                      }
                    }
                  }
                }
                frame "I16" {
                  # "Scaler type (so we are using the inlined function)"
                  n150 = case shown="3" w772 {
                    tunnel: [w778 w789 w808 w850] -> w777
                    tunnel: w776 -> [w778 w783 w806 w848]
                    tunnel: w775 -> [_ w788 w812 w854]
                    tunnel: [w779 w786 w810 w852] -> w774
                    tunnel: w770 -> [_ w785 w809 w851]
                    tunnel: w773 -> [_ w780 w804 w846]
                    tunnel: w771 -> [w779 w781 _ _]
                    tunnel: w769 -> [_ w784 w807 w849]
                    frame 0, Default {
                    }
                    frame 1 {
                      n151 = call "Get Array Elements (by Offset).vi"("error in (no error)"=w783, "Offset"=w785, "JSON"=w780) -> ("error out"=w782:errorcluster, "Element Offsets"=w787:i32[])  [unwired: 5 in, 2 out]
                      n152 = case shown="No Error" w782 {
                        selector: w782 -> [w791 w803]
                        tunnel: [w796 w803] -> w789
                        tunnel: w788 -> [w795 _]
                        tunnel: w787 -> [w794 _]
                        tunnel: [w793 _] -> w786
                        tunnel: w784 -> [w792 _]
                        tunnel: w781 -> [_ _]
                        tunnel: w780 -> [w790 _]
                        frame No Error {
                          n153 = for {
                            tunnel: w795 -> [_]
                            tunnel: [w798] -> w793 mode=indexing
                            tunnel: w794 -> [w799] mode=indexing
                            tunnel: w792 -> [_]
                            tunnel: w790 -> [w800]
                            shift-right: [w802] -> w796
                            shift-left: w791 -> [w801]
                            n154 = call "Get I16.vi"("Offset"=w799, "JSON"=w800) -> ("error out"=w797:errorcluster, "Number"=w798:i16)  [unwired: 7 in, 1 out]
                            n155 = Merge Errors(w801, w797) -> (w802:errorcluster)
                          }
                        }
                        frame Error {
                        }
                      }
                    }
                    frame 2 {
                      n156 = call "Get Array Elements (by Offset).vi"("error in (no error)"=w806, "Offset"=w809, "JSON"=w804) -> ("error out"=w805:errorcluster, "Element Offsets"=w811:i32[])  [unwired: 5 in, 2 out]
                      n157 = case shown="No Error" w805 {
                        selector: w805 -> [w815 w845]
                        tunnel: w812 -> [w819 _]
                        tunnel: w811 -> [w818 _]
                        tunnel: [w817 _] -> w810
                        tunnel: [w813 w845] -> w808
                        tunnel: w807 -> [w816 _]
                        tunnel: w804 -> [w814 _]
                        frame No Error {
                          n158 = for {
                            tunnel: w819 -> [w829]
                            tunnel: w818 -> [w824] mode=indexing
                            tunnel: [w828] -> w817 mode=indexing
                            tunnel: w816 -> [w826]
                            tunnel: w814 -> [w823]
                            tunnel: w814 -> [w822]
                            shift-right: [w821] -> w813
                            shift-left: w815 -> [w820]
                            n159 = call "Get Array Elements (by Offset).vi"("Offset"=w824, "JSON"=w823) -> ("error out"=w825:errorcluster, "Element Offsets"=w827:i32[])  [unwired: 6 in, 2 out]
                            n160 = case shown="No Error" w825 {
                              selector: w825 -> [w833 w844]
                              tunnel: [w831 w844] -> w830
                              tunnel: w829 -> [w837 _]
                              tunnel: [w836 _] -> w828
                              tunnel: w827 -> [w835 _]
                              tunnel: w826 -> [w834 _]
                              tunnel: w822 -> [w832 _]
                              frame No Error {
                                n161 = for {
                                tunnel: w837 -> [_]
                                tunnel: [w838] -> w836 mode=indexing
                                tunnel: w835 -> [w840] mode=indexing
                                tunnel: w834 -> [_]
                                tunnel: w832 -> [w841]
                                shift-right: [w843] -> w831
                                shift-left: w833 -> [w842]
                                n162 = call "Get I16.vi"("Offset"=w840, "JSON"=w841) -> ("error out"=w839:errorcluster, "Number"=w838:i16)  [unwired: 7 in, 1 out]
                                n163 = Merge Errors(w842, w839) -> (w843:errorcluster)
                                }
                              }
                              frame Error {
                              }
                            }
                            n164 = Merge Errors(w820, w830) -> (w821:errorcluster)
                          }
                        }
                        frame Error {
                        }
                      }
                    }
                    frame 3 {
                      n165 = call "Get Array Elements (by Offset).vi"("error in (no error)"=w848, "Offset"=w851, "JSON"=w846) -> ("error out"=w847:errorcluster, "Element Offsets"=w853:i32[])  [unwired: 5 in, 2 out]
                      n166 = case shown="No Error" w847 {
                        selector: w847 -> [w857 w907]
                        tunnel: w854 -> [w861 w906]
                        tunnel: w853 -> [w860 _]
                        tunnel: [w859 w906] -> w852
                        tunnel: [w855 w907] -> w850
                        tunnel: w849 -> [w858 _]
                        tunnel: w846 -> [w856 _]
                        frame No Error {
                          n167 = for {
                            tunnel: w861 -> [w871]
                            tunnel: w860 -> [w866] mode=indexing
                            tunnel: [w870] -> w859 mode=indexing
                            tunnel: w858 -> [w868]
                            tunnel: w856 -> [w865]
                            tunnel: w856 -> [w864]
                            shift-right: [w863] -> w855
                            shift-left: w857 -> [w862]
                            n168 = call "Get Array Elements (by Offset).vi"("Offset"=w866, "JSON"=w865) -> ("error out"=w867:errorcluster, "Element Offsets"=w869:i32[])  [unwired: 6 in, 2 out]
                            n169 = case shown="No Error" w867 {
                              selector: w867 -> [w873 w905]
                              tunnel: [w875 w905] -> w872
                              tunnel: w871 -> [w879 _]
                              tunnel: [w874 _] -> w870
                              tunnel: w869 -> [w878 _]
                              tunnel: w868 -> [w876 _]
                              tunnel: w864 -> [w877 _]
                              frame No Error {
                                n170 = for {
                                tunnel: w879 -> [w889]
                                tunnel: w878 -> [w884] mode=indexing
                                tunnel: [w888] -> w874 mode=indexing
                                tunnel: w876 -> [w886]
                                tunnel: w877 -> [w883]
                                tunnel: w877 -> [w882]
                                shift-right: [w881] -> w875
                                shift-left: w873 -> [w880]
                                n171 = call "Get Array Elements (by Offset).vi"("Offset"=w884, "JSON"=w883) -> ("error out"=w885:errorcluster, "Element Offsets"=w887:i32[])  [unwired: 6 in, 2 out]
                                n172 = case shown="No Error" w885 {
                                selector: w885 -> [w893 w904]
                                tunnel: [w891 w904] -> w890
                                tunnel: w889 -> [w897 _]
                                tunnel: [w896 _] -> w888
                                tunnel: w887 -> [w895 _]
                                tunnel: w886 -> [w894 _]
                                tunnel: w882 -> [w892 _]
                                frame No Error {
                                n173 = for {
                                tunnel: w897 -> [_]
                                tunnel: [w898] -> w896 mode=indexing
                                tunnel: w895 -> [w901] mode=indexing
                                tunnel: w894 -> [_]
                                tunnel: w892 -> [w902]
                                shift-right: [w903] -> w891
                                shift-left: w893 -> [w900]
                                n174 = call "Get I16.vi"("Offset"=w901, "JSON"=w902) -> ("error out"=w899:errorcluster, "Number"=w898:i16)  [unwired: 7 in, 1 out]
                                n175 = Merge Errors(w900, w899) -> (w903:errorcluster)
                                }
                                }
                                frame Error {
                                }
                                }
                                n176 = Merge Errors(w880, w890) -> (w881:errorcluster)
                                }
                              }
                              frame Error {
                              }
                            }
                            n177 = Merge Errors(w862, w872) -> (w863:errorcluster)
                          }
                        }
                        frame Error {
                        }
                      }
                    }
                  }
                }
                frame "I32" {
                  # "Scaler type (so we are using the inlined function)"
                  n178 = case shown="1" w911 {
                    tunnel: [w917 w928 w947 w989] -> w916
                    tunnel: w915 -> [w917 w922 w945 w987]
                    tunnel: w914 -> [_ w927 w951 w993]
                    tunnel: [w918 w925 w949 w991] -> w913
                    tunnel: w909 -> [_ w924 w948 w990]
                    tunnel: w912 -> [_ w919 w943 w985]
                    tunnel: w910 -> [w918 w920 _ _]
                    tunnel: w908 -> [_ w923 w946 w988]
                    frame 0, Default {
                    }
                    frame 1 {
                      n179 = call "Get Array Elements (by Offset).vi"("error in (no error)"=w922, "Offset"=w924, "JSON"=w919) -> ("error out"=w921:errorcluster, "Element Offsets"=w926:i32[])  [unwired: 5 in, 2 out]
                      n180 = case shown="No Error" w921 {
                        selector: w921 -> [w930 w942]
                        tunnel: [w935 w942] -> w928
                        tunnel: w927 -> [w934 _]
                        tunnel: w926 -> [w933 _]
                        tunnel: [w932 _] -> w925
                        tunnel: w923 -> [w931 _]
                        tunnel: w920 -> [_ _]
                        tunnel: w919 -> [w929 _]
                        frame No Error {
                          n181 = for {
                            tunnel: w934 -> [_]
                            tunnel: [w937] -> w932 mode=indexing
                            tunnel: w933 -> [w938] mode=indexing
                            tunnel: w931 -> [_]
                            tunnel: w929 -> [w939]
                            shift-right: [w941] -> w935
                            shift-left: w930 -> [w940]
                            n182 = call "Get I32.vi"("Offset"=w938, "JSON"=w939) -> ("error out"=w936:errorcluster, "Number"=w937:i32)  [unwired: 7 in, 1 out]
                            n183 = Merge Errors(w940, w936) -> (w941:errorcluster)
                          }
                        }
                        frame Error {
                        }
                      }
                    }
                    frame 2 {
                      n184 = call "Get Array Elements (by Offset).vi"("error in (no error)"=w945, "Offset"=w948, "JSON"=w943) -> ("error out"=w944:errorcluster, "Element Offsets"=w950:i32[])  [unwired: 5 in, 2 out]
                      n185 = case shown="No Error" w944 {
                        selector: w944 -> [w954 w984]
                        tunnel: w951 -> [w958 _]
                        tunnel: w950 -> [w957 _]
                        tunnel: [w956 _] -> w949
                        tunnel: [w952 w984] -> w947
                        tunnel: w946 -> [w955 _]
                        tunnel: w943 -> [w953 _]
                        frame No Error {
                          n186 = for {
                            tunnel: w958 -> [w968]
                            tunnel: w957 -> [w963] mode=indexing
                            tunnel: [w967] -> w956 mode=indexing
                            tunnel: w955 -> [w965]
                            tunnel: w953 -> [w962]
                            tunnel: w953 -> [w961]
                            shift-right: [w960] -> w952
                            shift-left: w954 -> [w959]
                            n187 = call "Get Array Elements (by Offset).vi"("Offset"=w963, "JSON"=w962) -> ("error out"=w964:errorcluster, "Element Offsets"=w966:i32[])  [unwired: 6 in, 2 out]
                            n188 = case shown="No Error" w964 {
                              selector: w964 -> [w972 w983]
                              tunnel: [w970 w983] -> w969
                              tunnel: w968 -> [w976 _]
                              tunnel: [w975 _] -> w967
                              tunnel: w966 -> [w974 _]
                              tunnel: w965 -> [w973 _]
                              tunnel: w961 -> [w971 _]
                              frame No Error {
                                n189 = for {
                                tunnel: w976 -> [_]
                                tunnel: [w977] -> w975 mode=indexing
                                tunnel: w974 -> [w979] mode=indexing
                                tunnel: w973 -> [_]
                                tunnel: w971 -> [w980]
                                shift-right: [w982] -> w970
                                shift-left: w972 -> [w981]
                                n190 = call "Get I32.vi"("Offset"=w979, "JSON"=w980) -> ("error out"=w978:errorcluster, "Number"=w977:i32)  [unwired: 7 in, 1 out]
                                n191 = Merge Errors(w981, w978) -> (w982:errorcluster)
                                }
                              }
                              frame Error {
                              }
                            }
                            n192 = Merge Errors(w959, w969) -> (w960:errorcluster)
                          }
                        }
                        frame Error {
                        }
                      }
                    }
                    frame 3 {
                      n193 = call "Get Array Elements (by Offset).vi"("error in (no error)"=w987, "Offset"=w990, "JSON"=w985) -> ("error out"=w986:errorcluster, "Element Offsets"=w992:i32[])  [unwired: 5 in, 2 out]
                      n194 = case shown="No Error" w986 {
                        selector: w986 -> [w996 w1046]
                        tunnel: w993 -> [w1000 w1045]
                        tunnel: w992 -> [w999 _]
                        tunnel: [w998 w1045] -> w991
                        tunnel: [w994 w1046] -> w989
                        tunnel: w988 -> [w997 _]
                        tunnel: w985 -> [w995 _]
                        frame No Error {
                          n195 = for {
                            tunnel: w1000 -> [w1010]
                            tunnel: w999 -> [w1005] mode=indexing
                            tunnel: [w1009] -> w998 mode=indexing
                            tunnel: w997 -> [w1007]
                            tunnel: w995 -> [w1004]
                            tunnel: w995 -> [w1003]
                            shift-right: [w1002] -> w994
                            shift-left: w996 -> [w1001]
                            n196 = call "Get Array Elements (by Offset).vi"("Offset"=w1005, "JSON"=w1004) -> ("error out"=w1006:errorcluster, "Element Offsets"=w1008:i32[])  [unwired: 6 in, 2 out]
                            n197 = case shown="No Error" w1006 {
                              selector: w1006 -> [w1012 w1044]
                              tunnel: [w1014 w1044] -> w1011
                              tunnel: w1010 -> [w1018 _]
                              tunnel: [w1013 _] -> w1009
                              tunnel: w1008 -> [w1017 _]
                              tunnel: w1007 -> [w1015 _]
                              tunnel: w1003 -> [w1016 _]
                              frame No Error {
                                n198 = for {
                                tunnel: w1018 -> [w1028]
                                tunnel: w1017 -> [w1023] mode=indexing
                                tunnel: [w1027] -> w1013 mode=indexing
                                tunnel: w1015 -> [w1025]
                                tunnel: w1016 -> [w1022]
                                tunnel: w1016 -> [w1021]
                                shift-right: [w1020] -> w1014
                                shift-left: w1012 -> [w1019]
                                n199 = call "Get Array Elements (by Offset).vi"("Offset"=w1023, "JSON"=w1022) -> ("error out"=w1024:errorcluster, "Element Offsets"=w1026:i32[])  [unwired: 6 in, 2 out]
                                n200 = case shown="No Error" w1024 {
                                selector: w1024 -> [w1032 w1043]
                                tunnel: [w1030 w1043] -> w1029
                                tunnel: w1028 -> [w1036 _]
                                tunnel: [w1035 _] -> w1027
                                tunnel: w1026 -> [w1034 _]
                                tunnel: w1025 -> [w1033 _]
                                tunnel: w1021 -> [w1031 _]
                                frame No Error {
                                n201 = for {
                                tunnel: w1036 -> [_]
                                tunnel: [w1037] -> w1035 mode=indexing
                                tunnel: w1034 -> [w1040] mode=indexing
                                tunnel: w1033 -> [_]
                                tunnel: w1031 -> [w1041]
                                shift-right: [w1042] -> w1030
                                shift-left: w1032 -> [w1039]
                                n202 = call "Get I32.vi"("Offset"=w1040, "JSON"=w1041) -> ("error out"=w1038:errorcluster, "Number"=w1037:i32)  [unwired: 7 in, 1 out]
                                n203 = Merge Errors(w1039, w1038) -> (w1042:errorcluster)
                                }
                                }
                                frame Error {
                                }
                                }
                                n204 = Merge Errors(w1019, w1029) -> (w1020:errorcluster)
                                }
                              }
                              frame Error {
                              }
                            }
                            n205 = Merge Errors(w1001, w1011) -> (w1002:errorcluster)
                          }
                        }
                        frame Error {
                        }
                      }
                    }
                  }
                }
                frame "I64" {
                  # "Scaler type (so we are using the inlined function)"
                  n206 = case shown="3" w1050 {
                    tunnel: [w1056 w1067 w1086 w1128] -> w1055
                    tunnel: w1054 -> [w1056 w1061 w1084 w1126]
                    tunnel: w1053 -> [_ w1066 w1090 w1132]
                    tunnel: [w1057 w1064 w1088 w1130] -> w1052
                    tunnel: w1048 -> [_ w1063 w1087 w1129]
                    tunnel: w1051 -> [_ w1058 w1082 w1124]
                    tunnel: w1049 -> [w1057 w1059 _ _]
                    tunnel: w1047 -> [_ w1062 w1085 w1127]
                    frame 0, Default {
                    }
                    frame 1 {
                      n207 = call "Get Array Elements (by Offset).vi"("error in (no error)"=w1061, "Offset"=w1063, "JSON"=w1058) -> ("error out"=w1060:errorcluster, "Element Offsets"=w1065:i32[])  [unwired: 5 in, 2 out]
                      n208 = case shown="No Error" w1060 {
                        selector: w1060 -> [w1069 w1081]
                        tunnel: [w1074 w1081] -> w1067
                        tunnel: w1066 -> [w1073 _]
                        tunnel: w1065 -> [w1072 _]
                        tunnel: [w1071 _] -> w1064
                        tunnel: w1062 -> [w1070 _]
                        tunnel: w1059 -> [_ _]
                        tunnel: w1058 -> [w1068 _]
                        frame No Error {
                          n209 = for {
                            tunnel: w1073 -> [_]
                            tunnel: [w1076] -> w1071 mode=indexing
                            tunnel: w1072 -> [w1077] mode=indexing
                            tunnel: w1070 -> [_]
                            tunnel: w1068 -> [w1078]
                            shift-right: [w1080] -> w1074
                            shift-left: w1069 -> [w1079]
                            n210 = call "Get I64.vi"("Offset"=w1077, "JSON"=w1078) -> ("error out"=w1075:errorcluster, "Number"=w1076:i64)  [unwired: 7 in, 1 out]
                            n211 = Merge Errors(w1079, w1075) -> (w1080:errorcluster)
                          }
                        }
                        frame Error {
                        }
                      }
                    }
                    frame 2 {
                      n212 = call "Get Array Elements (by Offset).vi"("error in (no error)"=w1084, "Offset"=w1087, "JSON"=w1082) -> ("error out"=w1083:errorcluster, "Element Offsets"=w1089:i32[])  [unwired: 5 in, 2 out]
                      n213 = case shown="No Error" w1083 {
                        selector: w1083 -> [w1093 w1123]
                        tunnel: w1090 -> [w1097 _]
                        tunnel: w1089 -> [w1096 _]
                        tunnel: [w1095 _] -> w1088
                        tunnel: [w1091 w1123] -> w1086
                        tunnel: w1085 -> [w1094 _]
                        tunnel: w1082 -> [w1092 _]
                        frame No Error {
                          n214 = for {
                            tunnel: w1097 -> [w1107]
                            tunnel: w1096 -> [w1102] mode=indexing
                            tunnel: [w1106] -> w1095 mode=indexing
                            tunnel: w1094 -> [w1104]
                            tunnel: w1092 -> [w1101]
                            tunnel: w1092 -> [w1100]
                            shift-right: [w1099] -> w1091
                            shift-left: w1093 -> [w1098]
                            n215 = call "Get Array Elements (by Offset).vi"("Offset"=w1102, "JSON"=w1101) -> ("error out"=w1103:errorcluster, "Element Offsets"=w1105:i32[])  [unwired: 6 in, 2 out]
                            n216 = case shown="No Error" w1103 {
                              selector: w1103 -> [w1111 w1122]
                              tunnel: [w1109 w1122] -> w1108
                              tunnel: w1107 -> [w1115 _]
                              tunnel: [w1114 _] -> w1106
                              tunnel: w1105 -> [w1113 _]
                              tunnel: w1104 -> [w1112 _]
                              tunnel: w1100 -> [w1110 _]
                              frame No Error {
                                n217 = for {
                                tunnel: w1115 -> [_]
                                tunnel: [w1116] -> w1114 mode=indexing
                                tunnel: w1113 -> [w1118] mode=indexing
                                tunnel: w1112 -> [_]
                                tunnel: w1110 -> [w1119]
                                shift-right: [w1121] -> w1109
                                shift-left: w1111 -> [w1120]
                                n218 = call "Get I64.vi"("Offset"=w1118, "JSON"=w1119) -> ("error out"=w1117:errorcluster, "Number"=w1116:i64)  [unwired: 7 in, 1 out]
                                n219 = Merge Errors(w1120, w1117) -> (w1121:errorcluster)
                                }
                              }
                              frame Error {
                              }
                            }
                            n220 = Merge Errors(w1098, w1108) -> (w1099:errorcluster)
                          }
                        }
                        frame Error {
                        }
                      }
                    }
                    frame 3 {
                      n221 = call "Get Array Elements (by Offset).vi"("error in (no error)"=w1126, "Offset"=w1129, "JSON"=w1124) -> ("error out"=w1125:errorcluster, "Element Offsets"=w1131:i32[])  [unwired: 5 in, 2 out]
                      n222 = case shown="No Error" w1125 {
                        selector: w1125 -> [w1135 w1185]
                        tunnel: w1132 -> [w1139 w1184]
                        tunnel: w1131 -> [w1138 _]
                        tunnel: [w1137 w1184] -> w1130
                        tunnel: [w1133 w1185] -> w1128
                        tunnel: w1127 -> [w1136 _]
                        tunnel: w1124 -> [w1134 _]
                        frame No Error {
                          n223 = for {
                            tunnel: w1139 -> [w1149]
                            tunnel: w1138 -> [w1144] mode=indexing
                            tunnel: [w1148] -> w1137 mode=indexing
                            tunnel: w1136 -> [w1146]
                            tunnel: w1134 -> [w1143]
                            tunnel: w1134 -> [w1142]
                            shift-right: [w1141] -> w1133
                            shift-left: w1135 -> [w1140]
                            n224 = call "Get Array Elements (by Offset).vi"("Offset"=w1144, "JSON"=w1143) -> ("error out"=w1145:errorcluster, "Element Offsets"=w1147:i32[])  [unwired: 6 in, 2 out]
                            n225 = case shown="No Error" w1145 {
                              selector: w1145 -> [w1151 w1183]
                              tunnel: [w1153 w1183] -> w1150
                              tunnel: w1149 -> [w1157 _]
                              tunnel: [w1152 _] -> w1148
                              tunnel: w1147 -> [w1156 _]
                              tunnel: w1146 -> [w1154 _]
                              tunnel: w1142 -> [w1155 _]
                              frame No Error {
                                n226 = for {
                                tunnel: w1157 -> [w1167]
                                tunnel: w1156 -> [w1162] mode=indexing
                                tunnel: [w1166] -> w1152 mode=indexing
                                tunnel: w1154 -> [w1164]
                                tunnel: w1155 -> [w1161]
                                tunnel: w1155 -> [w1160]
                                shift-right: [w1159] -> w1153
                                shift-left: w1151 -> [w1158]
                                n227 = call "Get Array Elements (by Offset).vi"("Offset"=w1162, "JSON"=w1161) -> ("error out"=w1163:errorcluster, "Element Offsets"=w1165:i32[])  [unwired: 6 in, 2 out]
                                n228 = case shown="No Error" w1163 {
                                selector: w1163 -> [w1171 w1182]
                                tunnel: [w1169 w1182] -> w1168
                                tunnel: w1167 -> [w1175 _]
                                tunnel: [w1174 _] -> w1166
                                tunnel: w1165 -> [w1173 _]
                                tunnel: w1164 -> [w1172 _]
                                tunnel: w1160 -> [w1170 _]
                                frame No Error {
                                n229 = for {
                                tunnel: w1175 -> [_]
                                tunnel: [w1176] -> w1174 mode=indexing
                                tunnel: w1173 -> [w1179] mode=indexing
                                tunnel: w1172 -> [_]
                                tunnel: w1170 -> [w1180]
                                shift-right: [w1181] -> w1169
                                shift-left: w1171 -> [w1178]
                                n230 = call "Get I64.vi"("Offset"=w1179, "JSON"=w1180) -> ("error out"=w1177:errorcluster, "Number"=w1176:i64)  [unwired: 7 in, 1 out]
                                n231 = Merge Errors(w1178, w1177) -> (w1181:errorcluster)
                                }
                                }
                                frame Error {
                                }
                                }
                                n232 = Merge Errors(w1158, w1168) -> (w1159:errorcluster)
                                }
                              }
                              frame Error {
                              }
                            }
                            n233 = Merge Errors(w1140, w1150) -> (w1141:errorcluster)
                          }
                        }
                        frame Error {
                        }
                      }
                    }
                  }
                }
                frame "U8" {
                  # "Scaler type (so we are using the inlined function)"
                  n234 = case shown="3" w1189 {
                    tunnel: [w1195 w1206 w1225 w1267] -> w1194
                    tunnel: w1193 -> [w1195 w1200 w1223 w1265]
                    tunnel: w1192 -> [_ w1205 w1229 w1271]
                    tunnel: [w1196 w1203 w1227 w1269] -> w1191
                    tunnel: w1187 -> [_ w1202 w1226 w1268]
                    tunnel: w1190 -> [_ w1197 w1221 w1263]
                    tunnel: w1188 -> [w1196 w1198 _ _]
                    tunnel: w1186 -> [_ w1201 w1224 w1266]
                    frame 0, Default {
                    }
                    frame 1 {
                      n235 = call "Get Array Elements (by Offset).vi"("error in (no error)"=w1200, "Offset"=w1202, "JSON"=w1197) -> ("error out"=w1199:errorcluster, "Element Offsets"=w1204:i32[])  [unwired: 5 in, 2 out]
                      n236 = case shown="No Error" w1199 {
                        selector: w1199 -> [w1208 w1220]
                        tunnel: [w1213 w1220] -> w1206
                        tunnel: w1205 -> [w1212 _]
                        tunnel: w1204 -> [w1211 _]
                        tunnel: [w1210 _] -> w1203
                        tunnel: w1201 -> [w1209 _]
                        tunnel: w1198 -> [_ _]
                        tunnel: w1197 -> [w1207 _]
                        frame No Error {
                          n237 = for {
                            tunnel: w1212 -> [_]
                            tunnel: [w1215] -> w1210 mode=indexing
                            tunnel: w1211 -> [w1216] mode=indexing
                            tunnel: w1209 -> [_]
                            tunnel: w1207 -> [w1217]
                            shift-right: [w1219] -> w1213
                            shift-left: w1208 -> [w1218]
                            n238 = call "Get U8.vi"("Offset"=w1216, "JSON"=w1217) -> ("error out"=w1214:errorcluster, "Number"=w1215:u8)  [unwired: 7 in, 1 out]
                            n239 = Merge Errors(w1218, w1214) -> (w1219:errorcluster)
                          }
                        }
                        frame Error {
                        }
                      }
                    }
                    frame 2 {
                      n240 = call "Get Array Elements (by Offset).vi"("error in (no error)"=w1223, "Offset"=w1226, "JSON"=w1221) -> ("error out"=w1222:errorcluster, "Element Offsets"=w1228:i32[])  [unwired: 5 in, 2 out]
                      n241 = case shown="No Error" w1222 {
                        selector: w1222 -> [w1232 w1262]
                        tunnel: w1229 -> [w1236 _]
                        tunnel: w1228 -> [w1235 _]
                        tunnel: [w1234 _] -> w1227
                        tunnel: [w1230 w1262] -> w1225
                        tunnel: w1224 -> [w1233 _]
                        tunnel: w1221 -> [w1231 _]
                        frame No Error {
                          n242 = for {
                            tunnel: w1236 -> [w1246]
                            tunnel: w1235 -> [w1241] mode=indexing
                            tunnel: [w1245] -> w1234 mode=indexing
                            tunnel: w1233 -> [w1243]
                            tunnel: w1231 -> [w1240]
                            tunnel: w1231 -> [w1239]
                            shift-right: [w1238] -> w1230
                            shift-left: w1232 -> [w1237]
                            n243 = call "Get Array Elements (by Offset).vi"("Offset"=w1241, "JSON"=w1240) -> ("error out"=w1242:errorcluster, "Element Offsets"=w1244:i32[])  [unwired: 6 in, 2 out]
                            n244 = case shown="No Error" w1242 {
                              selector: w1242 -> [w1250 w1261]
                              tunnel: [w1248 w1261] -> w1247
                              tunnel: w1246 -> [w1254 _]
                              tunnel: [w1253 _] -> w1245
                              tunnel: w1244 -> [w1252 _]
                              tunnel: w1243 -> [w1251 _]
                              tunnel: w1239 -> [w1249 _]
                              frame No Error {
                                n245 = for {
                                tunnel: w1254 -> [_]
                                tunnel: [w1255] -> w1253 mode=indexing
                                tunnel: w1252 -> [w1257] mode=indexing
                                tunnel: w1251 -> [_]
                                tunnel: w1249 -> [w1258]
                                shift-right: [w1260] -> w1248
                                shift-left: w1250 -> [w1259]
                                n246 = call "Get U8.vi"("Offset"=w1257, "JSON"=w1258) -> ("error out"=w1256:errorcluster, "Number"=w1255:u8)  [unwired: 7 in, 1 out]
                                n247 = Merge Errors(w1259, w1256) -> (w1260:errorcluster)
                                }
                              }
                              frame Error {
                              }
                            }
                            n248 = Merge Errors(w1237, w1247) -> (w1238:errorcluster)
                          }
                        }
                        frame Error {
                        }
                      }
                    }
                    frame 3 {
                      n249 = call "Get Array Elements (by Offset).vi"("error in (no error)"=w1265, "Offset"=w1268, "JSON"=w1263) -> ("error out"=w1264:errorcluster, "Element Offsets"=w1270:i32[])  [unwired: 5 in, 2 out]
                      n250 = case shown="No Error" w1264 {
                        selector: w1264 -> [w1274 w1324]
                        tunnel: w1271 -> [w1278 w1323]
                        tunnel: w1270 -> [w1277 _]
                        tunnel: [w1276 w1323] -> w1269
                        tunnel: [w1272 w1324] -> w1267
                        tunnel: w1266 -> [w1275 _]
                        tunnel: w1263 -> [w1273 _]
                        frame No Error {
                          n251 = for {
                            tunnel: w1278 -> [w1288]
                            tunnel: w1277 -> [w1283] mode=indexing
                            tunnel: [w1287] -> w1276 mode=indexing
                            tunnel: w1275 -> [w1285]
                            tunnel: w1273 -> [w1282]
                            tunnel: w1273 -> [w1281]
                            shift-right: [w1280] -> w1272
                            shift-left: w1274 -> [w1279]
                            n252 = call "Get Array Elements (by Offset).vi"("Offset"=w1283, "JSON"=w1282) -> ("error out"=w1284:errorcluster, "Element Offsets"=w1286:i32[])  [unwired: 6 in, 2 out]
                            n253 = case shown="No Error" w1284 {
                              selector: w1284 -> [w1290 w1322]
                              tunnel: [w1292 w1322] -> w1289
                              tunnel: w1288 -> [w1296 _]
                              tunnel: [w1291 _] -> w1287
                              tunnel: w1286 -> [w1295 _]
                              tunnel: w1285 -> [w1293 _]
                              tunnel: w1281 -> [w1294 _]
                              frame No Error {
                                n254 = for {
                                tunnel: w1296 -> [w1306]
                                tunnel: w1295 -> [w1301] mode=indexing
                                tunnel: [w1305] -> w1291 mode=indexing
                                tunnel: w1293 -> [w1303]
                                tunnel: w1294 -> [w1300]
                                tunnel: w1294 -> [w1299]
                                shift-right: [w1298] -> w1292
                                shift-left: w1290 -> [w1297]
                                n255 = call "Get Array Elements (by Offset).vi"("Offset"=w1301, "JSON"=w1300) -> ("error out"=w1302:errorcluster, "Element Offsets"=w1304:i32[])  [unwired: 6 in, 2 out]
                                n256 = case shown="No Error" w1302 {
                                selector: w1302 -> [w1310 w1321]
                                tunnel: [w1308 w1321] -> w1307
                                tunnel: w1306 -> [w1314 _]
                                tunnel: [w1313 _] -> w1305
                                tunnel: w1304 -> [w1312 _]
                                tunnel: w1303 -> [w1311 _]
                                tunnel: w1299 -> [w1309 _]
                                frame No Error {
                                n257 = for {
                                tunnel: w1314 -> [_]
                                tunnel: [w1315] -> w1313 mode=indexing
                                tunnel: w1312 -> [w1318] mode=indexing
                                tunnel: w1311 -> [_]
                                tunnel: w1309 -> [w1319]
                                shift-right: [w1320] -> w1308
                                shift-left: w1310 -> [w1317]
                                n258 = call "Get U8.vi"("Offset"=w1318, "JSON"=w1319) -> ("error out"=w1316:errorcluster, "Number"=w1315:u8)  [unwired: 7 in, 1 out]
                                n259 = Merge Errors(w1317, w1316) -> (w1320:errorcluster)
                                }
                                }
                                frame Error {
                                }
                                }
                                n260 = Merge Errors(w1297, w1307) -> (w1298:errorcluster)
                                }
                              }
                              frame Error {
                              }
                            }
                            n261 = Merge Errors(w1279, w1289) -> (w1280:errorcluster)
                          }
                        }
                        frame Error {
                        }
                      }
                    }
                  }
                }
                frame "U16" {
                  # "Scaler type (so we are using the inlined function)"
                  n262 = case shown="3" w1328 {
                    tunnel: [w1334 w1345 w1364 w1406] -> w1333
                    tunnel: w1332 -> [w1334 w1339 w1362 w1404]
                    tunnel: w1331 -> [_ w1344 w1368 w1410]
                    tunnel: [w1335 w1342 w1366 w1408] -> w1330
                    tunnel: w1326 -> [_ w1341 w1365 w1407]
                    tunnel: w1329 -> [_ w1336 w1360 w1402]
                    tunnel: w1327 -> [w1335 w1337 _ _]
                    tunnel: w1325 -> [_ w1340 w1363 w1405]
                    frame 0, Default {
                    }
                    frame 1 {
                      n263 = call "Get Array Elements (by Offset).vi"("error in (no error)"=w1339, "Offset"=w1341, "JSON"=w1336) -> ("error out"=w1338:errorcluster, "Element Offsets"=w1343:i32[])  [unwired: 5 in, 2 out]
                      n264 = case shown="No Error" w1338 {
                        selector: w1338 -> [w1347 w1359]
                        tunnel: [w1352 w1359] -> w1345
                        tunnel: w1344 -> [w1351 _]
                        tunnel: w1343 -> [w1350 _]
                        tunnel: [w1349 _] -> w1342
                        tunnel: w1340 -> [w1348 _]
                        tunnel: w1337 -> [_ _]
                        tunnel: w1336 -> [w1346 _]
                        frame No Error {
                          n265 = for {
                            tunnel: w1351 -> [_]
                            tunnel: [w1354] -> w1349 mode=indexing
                            tunnel: w1350 -> [w1355] mode=indexing
                            tunnel: w1348 -> [_]
                            tunnel: w1346 -> [w1356]
                            shift-right: [w1358] -> w1352
                            shift-left: w1347 -> [w1357]
                            n266 = call "Get U16.vi"("Offset"=w1355, "JSON"=w1356) -> ("error out"=w1353:errorcluster, "Number"=w1354:u16)  [unwired: 7 in, 1 out]
                            n267 = Merge Errors(w1357, w1353) -> (w1358:errorcluster)
                          }
                        }
                        frame Error {
                        }
                      }
                    }
                    frame 2 {
                      n268 = call "Get Array Elements (by Offset).vi"("error in (no error)"=w1362, "Offset"=w1365, "JSON"=w1360) -> ("error out"=w1361:errorcluster, "Element Offsets"=w1367:i32[])  [unwired: 5 in, 2 out]
                      n269 = case shown="No Error" w1361 {
                        selector: w1361 -> [w1371 w1401]
                        tunnel: w1368 -> [w1375 _]
                        tunnel: w1367 -> [w1374 _]
                        tunnel: [w1373 _] -> w1366
                        tunnel: [w1369 w1401] -> w1364
                        tunnel: w1363 -> [w1372 _]
                        tunnel: w1360 -> [w1370 _]
                        frame No Error {
                          n270 = for {
                            tunnel: w1375 -> [w1385]
                            tunnel: w1374 -> [w1380] mode=indexing
                            tunnel: [w1384] -> w1373 mode=indexing
                            tunnel: w1372 -> [w1382]
                            tunnel: w1370 -> [w1379]
                            tunnel: w1370 -> [w1378]
                            shift-right: [w1377] -> w1369
                            shift-left: w1371 -> [w1376]
                            n271 = call "Get Array Elements (by Offset).vi"("Offset"=w1380, "JSON"=w1379) -> ("error out"=w1381:errorcluster, "Element Offsets"=w1383:i32[])  [unwired: 6 in, 2 out]
                            n272 = case shown="No Error" w1381 {
                              selector: w1381 -> [w1389 w1400]
                              tunnel: [w1387 w1400] -> w1386
                              tunnel: w1385 -> [w1393 _]
                              tunnel: [w1392 _] -> w1384
                              tunnel: w1383 -> [w1391 _]
                              tunnel: w1382 -> [w1390 _]
                              tunnel: w1378 -> [w1388 _]
                              frame No Error {
                                n273 = for {
                                tunnel: w1393 -> [_]
                                tunnel: [w1394] -> w1392 mode=indexing
                                tunnel: w1391 -> [w1396] mode=indexing
                                tunnel: w1390 -> [_]
                                tunnel: w1388 -> [w1397]
                                shift-right: [w1399] -> w1387
                                shift-left: w1389 -> [w1398]
                                n274 = call "Get U16.vi"("Offset"=w1396, "JSON"=w1397) -> ("error out"=w1395:errorcluster, "Number"=w1394:u16)  [unwired: 7 in, 1 out]
                                n275 = Merge Errors(w1398, w1395) -> (w1399:errorcluster)
                                }
                              }
                              frame Error {
                              }
                            }
                            n276 = Merge Errors(w1376, w1386) -> (w1377:errorcluster)
                          }
                        }
                        frame Error {
                        }
                      }
                    }
                    frame 3 {
                      n277 = call "Get Array Elements (by Offset).vi"("error in (no error)"=w1404, "Offset"=w1407, "JSON"=w1402) -> ("error out"=w1403:errorcluster, "Element Offsets"=w1409:i32[])  [unwired: 5 in, 2 out]
                      n278 = case shown="No Error" w1403 {
                        selector: w1403 -> [w1413 w1463]
                        tunnel: w1410 -> [w1417 w1462]
                        tunnel: w1409 -> [w1416 _]
                        tunnel: [w1415 w1462] -> w1408
                        tunnel: [w1411 w1463] -> w1406
                        tunnel: w1405 -> [w1414 _]
                        tunnel: w1402 -> [w1412 _]
                        frame No Error {
                          n279 = for {
                            tunnel: w1417 -> [w1427]
                            tunnel: w1416 -> [w1422] mode=indexing
                            tunnel: [w1426] -> w1415 mode=indexing
                            tunnel: w1414 -> [w1424]
                            tunnel: w1412 -> [w1421]
                            tunnel: w1412 -> [w1420]
                            shift-right: [w1419] -> w1411
                            shift-left: w1413 -> [w1418]
                            n280 = call "Get Array Elements (by Offset).vi"("Offset"=w1422, "JSON"=w1421) -> ("error out"=w1423:errorcluster, "Element Offsets"=w1425:i32[])  [unwired: 6 in, 2 out]
                            n281 = case shown="No Error" w1423 {
                              selector: w1423 -> [w1429 w1461]
                              tunnel: [w1431 w1461] -> w1428
                              tunnel: w1427 -> [w1435 _]
                              tunnel: [w1430 _] -> w1426
                              tunnel: w1425 -> [w1434 _]
                              tunnel: w1424 -> [w1432 _]
                              tunnel: w1420 -> [w1433 _]
                              frame No Error {
                                n282 = for {
                                tunnel: w1435 -> [w1445]
                                tunnel: w1434 -> [w1440] mode=indexing
                                tunnel: [w1444] -> w1430 mode=indexing
                                tunnel: w1432 -> [w1442]
                                tunnel: w1433 -> [w1439]
                                tunnel: w1433 -> [w1438]
                                shift-right: [w1437] -> w1431
                                shift-left: w1429 -> [w1436]
                                n283 = call "Get Array Elements (by Offset).vi"("Offset"=w1440, "JSON"=w1439) -> ("error out"=w1441:errorcluster, "Element Offsets"=w1443:i32[])  [unwired: 6 in, 2 out]
                                n284 = case shown="No Error" w1441 {
                                selector: w1441 -> [w1449 w1460]
                                tunnel: [w1447 w1460] -> w1446
                                tunnel: w1445 -> [w1453 _]
                                tunnel: [w1452 _] -> w1444
                                tunnel: w1443 -> [w1451 _]
                                tunnel: w1442 -> [w1450 _]
                                tunnel: w1438 -> [w1448 _]
                                frame No Error {
                                n285 = for {
                                tunnel: w1453 -> [_]
                                tunnel: [w1454] -> w1452 mode=indexing
                                tunnel: w1451 -> [w1457] mode=indexing
                                tunnel: w1450 -> [_]
                                tunnel: w1448 -> [w1458]
                                shift-right: [w1459] -> w1447
                                shift-left: w1449 -> [w1456]
                                n286 = call "Get U16.vi"("Offset"=w1457, "JSON"=w1458) -> ("error out"=w1455:errorcluster, "Number"=w1454:u16)  [unwired: 7 in, 1 out]
                                n287 = Merge Errors(w1456, w1455) -> (w1459:errorcluster)
                                }
                                }
                                frame Error {
                                }
                                }
                                n288 = Merge Errors(w1436, w1446) -> (w1437:errorcluster)
                                }
                              }
                              frame Error {
                              }
                            }
                            n289 = Merge Errors(w1418, w1428) -> (w1419:errorcluster)
                          }
                        }
                        frame Error {
                        }
                      }
                    }
                  }
                }
                frame "U32" {
                  # "Scaler type (so we are using the inlined function)"
                  n290 = case shown="3" w1467 {
                    tunnel: [w1473 w1484 w1503 w1545] -> w1472
                    tunnel: w1471 -> [w1473 w1478 w1501 w1543]
                    tunnel: w1470 -> [_ w1483 w1507 w1549]
                    tunnel: [w1474 w1481 w1505 w1547] -> w1469
                    tunnel: w1465 -> [_ w1480 w1504 w1546]
                    tunnel: w1468 -> [_ w1475 w1499 w1541]
                    tunnel: w1466 -> [w1474 w1476 _ _]
                    tunnel: w1464 -> [_ w1479 w1502 w1544]
                    frame 0, Default {
                    }
                    frame 1 {
                      n291 = call "Get Array Elements (by Offset).vi"("error in (no error)"=w1478, "Offset"=w1480, "JSON"=w1475) -> ("error out"=w1477:errorcluster, "Element Offsets"=w1482:i32[])  [unwired: 5 in, 2 out]
                      n292 = case shown="No Error" w1477 {
                        selector: w1477 -> [w1486 w1498]
                        tunnel: [w1491 w1498] -> w1484
                        tunnel: w1483 -> [w1490 _]
                        tunnel: w1482 -> [w1489 _]
                        tunnel: [w1488 _] -> w1481
                        tunnel: w1479 -> [w1487 _]
                        tunnel: w1476 -> [_ _]
                        tunnel: w1475 -> [w1485 _]
                        frame No Error {
                          n293 = for {
                            tunnel: w1490 -> [_]
                            tunnel: [w1493] -> w1488 mode=indexing
                            tunnel: w1489 -> [w1494] mode=indexing
                            tunnel: w1487 -> [_]
                            tunnel: w1485 -> [w1495]
                            shift-right: [w1497] -> w1491
                            shift-left: w1486 -> [w1496]
                            n294 = call "Get U32.vi"("Offset"=w1494, "JSON"=w1495) -> ("error out"=w1492:errorcluster, "Number"=w1493:u32)  [unwired: 7 in, 1 out]
                            n295 = Merge Errors(w1496, w1492) -> (w1497:errorcluster)
                          }
                        }
                        frame Error {
                        }
                      }
                    }
                    frame 2 {
                      n296 = call "Get Array Elements (by Offset).vi"("error in (no error)"=w1501, "Offset"=w1504, "JSON"=w1499) -> ("error out"=w1500:errorcluster, "Element Offsets"=w1506:i32[])  [unwired: 5 in, 2 out]
                      n297 = case shown="No Error" w1500 {
                        selector: w1500 -> [w1510 w1540]
                        tunnel: w1507 -> [w1514 _]
                        tunnel: w1506 -> [w1513 _]
                        tunnel: [w1512 _] -> w1505
                        tunnel: [w1508 w1540] -> w1503
                        tunnel: w1502 -> [w1511 _]
                        tunnel: w1499 -> [w1509 _]
                        frame No Error {
                          n298 = for {
                            tunnel: w1514 -> [w1524]
                            tunnel: w1513 -> [w1519] mode=indexing
                            tunnel: [w1523] -> w1512 mode=indexing
                            tunnel: w1511 -> [w1521]
                            tunnel: w1509 -> [w1518]
                            tunnel: w1509 -> [w1517]
                            shift-right: [w1516] -> w1508
                            shift-left: w1510 -> [w1515]
                            n299 = call "Get Array Elements (by Offset).vi"("Offset"=w1519, "JSON"=w1518) -> ("error out"=w1520:errorcluster, "Element Offsets"=w1522:i32[])  [unwired: 6 in, 2 out]
                            n300 = case shown="No Error" w1520 {
                              selector: w1520 -> [w1528 w1539]
                              tunnel: [w1526 w1539] -> w1525
                              tunnel: w1524 -> [w1532 _]
                              tunnel: [w1531 _] -> w1523
                              tunnel: w1522 -> [w1530 _]
                              tunnel: w1521 -> [w1529 _]
                              tunnel: w1517 -> [w1527 _]
                              frame No Error {
                                n301 = for {
                                tunnel: w1532 -> [_]
                                tunnel: [w1533] -> w1531 mode=indexing
                                tunnel: w1530 -> [w1535] mode=indexing
                                tunnel: w1529 -> [_]
                                tunnel: w1527 -> [w1536]
                                shift-right: [w1538] -> w1526
                                shift-left: w1528 -> [w1537]
                                n302 = call "Get U32.vi"("Offset"=w1535, "JSON"=w1536) -> ("error out"=w1534:errorcluster, "Number"=w1533:u32)  [unwired: 7 in, 1 out]
                                n303 = Merge Errors(w1537, w1534) -> (w1538:errorcluster)
                                }
                              }
                              frame Error {
                              }
                            }
                            n304 = Merge Errors(w1515, w1525) -> (w1516:errorcluster)
                          }
                        }
                        frame Error {
                        }
                      }
                    }
                    frame 3 {
                      n305 = call "Get Array Elements (by Offset).vi"("error in (no error)"=w1543, "Offset"=w1546, "JSON"=w1541) -> ("error out"=w1542:errorcluster, "Element Offsets"=w1548:i32[])  [unwired: 5 in, 2 out]
                      n306 = case shown="No Error" w1542 {
                        selector: w1542 -> [w1552 w1602]
                        tunnel: w1549 -> [w1556 w1601]
                        tunnel: w1548 -> [w1555 _]
                        tunnel: [w1554 w1601] -> w1547
                        tunnel: [w1550 w1602] -> w1545
                        tunnel: w1544 -> [w1553 _]
                        tunnel: w1541 -> [w1551 _]
                        frame No Error {
                          n307 = for {
                            tunnel: w1556 -> [w1566]
                            tunnel: w1555 -> [w1561] mode=indexing
                            tunnel: [w1565] -> w1554 mode=indexing
                            tunnel: w1553 -> [w1563]
                            tunnel: w1551 -> [w1560]
                            tunnel: w1551 -> [w1559]
                            shift-right: [w1558] -> w1550
                            shift-left: w1552 -> [w1557]
                            n308 = call "Get Array Elements (by Offset).vi"("Offset"=w1561, "JSON"=w1560) -> ("error out"=w1562:errorcluster, "Element Offsets"=w1564:i32[])  [unwired: 6 in, 2 out]
                            n309 = case shown="No Error" w1562 {
                              selector: w1562 -> [w1568 w1600]
                              tunnel: [w1570 w1600] -> w1567
                              tunnel: w1566 -> [w1574 _]
                              tunnel: [w1569 _] -> w1565
                              tunnel: w1564 -> [w1573 _]
                              tunnel: w1563 -> [w1571 _]
                              tunnel: w1559 -> [w1572 _]
                              frame No Error {
                                n310 = for {
                                tunnel: w1574 -> [w1584]
                                tunnel: w1573 -> [w1579] mode=indexing
                                tunnel: [w1583] -> w1569 mode=indexing
                                tunnel: w1571 -> [w1581]
                                tunnel: w1572 -> [w1578]
                                tunnel: w1572 -> [w1577]
                                shift-right: [w1576] -> w1570
                                shift-left: w1568 -> [w1575]
                                n311 = call "Get Array Elements (by Offset).vi"("Offset"=w1579, "JSON"=w1578) -> ("error out"=w1580:errorcluster, "Element Offsets"=w1582:i32[])  [unwired: 6 in, 2 out]
                                n312 = case shown="No Error" w1580 {
                                selector: w1580 -> [w1588 w1599]
                                tunnel: [w1586 w1599] -> w1585
                                tunnel: w1584 -> [w1592 _]
                                tunnel: [w1591 _] -> w1583
                                tunnel: w1582 -> [w1590 _]
                                tunnel: w1581 -> [w1589 _]
                                tunnel: w1577 -> [w1587 _]
                                frame No Error {
                                n313 = for {
                                tunnel: w1592 -> [_]
                                tunnel: [w1593] -> w1591 mode=indexing
                                tunnel: w1590 -> [w1596] mode=indexing
                                tunnel: w1589 -> [_]
                                tunnel: w1587 -> [w1597]
                                shift-right: [w1598] -> w1586
                                shift-left: w1588 -> [w1595]
                                n314 = call "Get U32.vi"("Offset"=w1596, "JSON"=w1597) -> ("error out"=w1594:errorcluster, "Number"=w1593:u32)  [unwired: 7 in, 1 out]
                                n315 = Merge Errors(w1595, w1594) -> (w1598:errorcluster)
                                }
                                }
                                frame Error {
                                }
                                }
                                n316 = Merge Errors(w1575, w1585) -> (w1576:errorcluster)
                                }
                              }
                              frame Error {
                              }
                            }
                            n317 = Merge Errors(w1557, w1567) -> (w1558:errorcluster)
                          }
                        }
                        frame Error {
                        }
                      }
                    }
                  }
                }
                frame "U64" {
                  # "Scaler type (so we are using the inlined function)"
                  n318 = case shown="3" w1606 {
                    tunnel: [w1612 w1623 w1642 w1684] -> w1611
                    tunnel: w1610 -> [w1612 w1617 w1640 w1682]
                    tunnel: w1609 -> [_ w1622 w1646 w1688]
                    tunnel: [w1613 w1620 w1644 w1686] -> w1608
                    tunnel: w1604 -> [_ w1619 w1643 w1685]
                    tunnel: w1607 -> [_ w1614 w1638 w1680]
                    tunnel: w1605 -> [w1613 w1615 _ _]
                    tunnel: w1603 -> [_ w1618 w1641 w1683]
                    frame 0, Default {
                    }
                    frame 1 {
                      n319 = call "Get Array Elements (by Offset).vi"("error in (no error)"=w1617, "Offset"=w1619, "JSON"=w1614) -> ("error out"=w1616:errorcluster, "Element Offsets"=w1621:i32[])  [unwired: 5 in, 2 out]
                      n320 = case shown="No Error" w1616 {
                        selector: w1616 -> [w1625 w1637]
                        tunnel: [w1630 w1637] -> w1623
                        tunnel: w1622 -> [w1629 _]
                        tunnel: w1621 -> [w1628 _]
                        tunnel: [w1627 _] -> w1620
                        tunnel: w1618 -> [w1626 _]
                        tunnel: w1615 -> [_ _]
                        tunnel: w1614 -> [w1624 _]
                        frame No Error {
                          n321 = for {
                            tunnel: w1629 -> [_]
                            tunnel: [w1632] -> w1627 mode=indexing
                            tunnel: w1628 -> [w1633] mode=indexing
                            tunnel: w1626 -> [_]
                            tunnel: w1624 -> [w1634]
                            shift-right: [w1636] -> w1630
                            shift-left: w1625 -> [w1635]
                            n322 = call "Get U64.vi"("Offset"=w1633, "JSON"=w1634) -> ("error out"=w1631:errorcluster, "Number"=w1632:u64)  [unwired: 7 in, 1 out]
                            n323 = Merge Errors(w1635, w1631) -> (w1636:errorcluster)
                          }
                        }
                        frame Error {
                        }
                      }
                    }
                    frame 2 {
                      n324 = call "Get Array Elements (by Offset).vi"("error in (no error)"=w1640, "Offset"=w1643, "JSON"=w1638) -> ("error out"=w1639:errorcluster, "Element Offsets"=w1645:i32[])  [unwired: 5 in, 2 out]
                      n325 = case shown="No Error" w1639 {
                        selector: w1639 -> [w1649 w1679]
                        tunnel: w1646 -> [w1653 _]
                        tunnel: w1645 -> [w1652 _]
                        tunnel: [w1651 _] -> w1644
                        tunnel: [w1647 w1679] -> w1642
                        tunnel: w1641 -> [w1650 _]
                        tunnel: w1638 -> [w1648 _]
                        frame No Error {
                          n326 = for {
                            tunnel: w1653 -> [w1663]
                            tunnel: w1652 -> [w1658] mode=indexing
                            tunnel: [w1662] -> w1651 mode=indexing
                            tunnel: w1650 -> [w1660]
                            tunnel: w1648 -> [w1657]
                            tunnel: w1648 -> [w1656]
                            shift-right: [w1655] -> w1647
                            shift-left: w1649 -> [w1654]
                            n327 = call "Get Array Elements (by Offset).vi"("Offset"=w1658, "JSON"=w1657) -> ("error out"=w1659:errorcluster, "Element Offsets"=w1661:i32[])  [unwired: 6 in, 2 out]
                            n328 = case shown="No Error" w1659 {
                              selector: w1659 -> [w1667 w1678]
                              tunnel: [w1665 w1678] -> w1664
                              tunnel: w1663 -> [w1671 _]
                              tunnel: [w1670 _] -> w1662
                              tunnel: w1661 -> [w1669 _]
                              tunnel: w1660 -> [w1668 _]
                              tunnel: w1656 -> [w1666 _]
                              frame No Error {
                                n329 = for {
                                tunnel: w1671 -> [_]
                                tunnel: [w1672] -> w1670 mode=indexing
                                tunnel: w1669 -> [w1674] mode=indexing
                                tunnel: w1668 -> [_]
                                tunnel: w1666 -> [w1675]
                                shift-right: [w1677] -> w1665
                                shift-left: w1667 -> [w1676]
                                n330 = call "Get U64.vi"("Offset"=w1674, "JSON"=w1675) -> ("error out"=w1673:errorcluster, "Number"=w1672:u64)  [unwired: 7 in, 1 out]
                                n331 = Merge Errors(w1676, w1673) -> (w1677:errorcluster)
                                }
                              }
                              frame Error {
                              }
                            }
                            n332 = Merge Errors(w1654, w1664) -> (w1655:errorcluster)
                          }
                        }
                        frame Error {
                        }
                      }
                    }
                    frame 3 {
                      n333 = call "Get Array Elements (by Offset).vi"("error in (no error)"=w1682, "Offset"=w1685, "JSON"=w1680) -> ("error out"=w1681:errorcluster, "Element Offsets"=w1687:i32[])  [unwired: 5 in, 2 out]
                      n334 = case shown="No Error" w1681 {
                        selector: w1681 -> [w1691 w1741]
                        tunnel: w1688 -> [w1695 w1740]
                        tunnel: w1687 -> [w1694 _]
                        tunnel: [w1693 w1740] -> w1686
                        tunnel: [w1689 w1741] -> w1684
                        tunnel: w1683 -> [w1692 _]
                        tunnel: w1680 -> [w1690 _]
                        frame No Error {
                          n335 = for {
                            tunnel: w1695 -> [w1705]
                            tunnel: w1694 -> [w1700] mode=indexing
                            tunnel: [w1704] -> w1693 mode=indexing
                            tunnel: w1692 -> [w1702]
                            tunnel: w1690 -> [w1699]
                            tunnel: w1690 -> [w1698]
                            shift-right: [w1697] -> w1689
                            shift-left: w1691 -> [w1696]
                            n336 = call "Get Array Elements (by Offset).vi"("Offset"=w1700, "JSON"=w1699) -> ("error out"=w1701:errorcluster, "Element Offsets"=w1703:i32[])  [unwired: 6 in, 2 out]
                            n337 = case shown="No Error" w1701 {
                              selector: w1701 -> [w1707 w1739]
                              tunnel: [w1709 w1739] -> w1706
                              tunnel: w1705 -> [w1713 _]
                              tunnel: [w1708 _] -> w1704
                              tunnel: w1703 -> [w1712 _]
                              tunnel: w1702 -> [w1710 _]
                              tunnel: w1698 -> [w1711 _]
                              frame No Error {
                                n338 = for {
                                tunnel: w1713 -> [w1723]
                                tunnel: w1712 -> [w1718] mode=indexing
                                tunnel: [w1722] -> w1708 mode=indexing
                                tunnel: w1710 -> [w1720]
                                tunnel: w1711 -> [w1717]
                                tunnel: w1711 -> [w1716]
                                shift-right: [w1715] -> w1709
                                shift-left: w1707 -> [w1714]
                                n339 = call "Get Array Elements (by Offset).vi"("Offset"=w1718, "JSON"=w1717) -> ("error out"=w1719:errorcluster, "Element Offsets"=w1721:i32[])  [unwired: 6 in, 2 out]
                                n340 = case shown="No Error" w1719 {
                                selector: w1719 -> [w1727 w1738]
                                tunnel: [w1725 w1738] -> w1724
                                tunnel: w1723 -> [w1731 _]
                                tunnel: [w1730 _] -> w1722
                                tunnel: w1721 -> [w1729 _]
                                tunnel: w1720 -> [w1728 _]
                                tunnel: w1716 -> [w1726 _]
                                frame No Error {
                                n341 = for {
                                tunnel: w1731 -> [_]
                                tunnel: [w1732] -> w1730 mode=indexing
                                tunnel: w1729 -> [w1735] mode=indexing
                                tunnel: w1728 -> [_]
                                tunnel: w1726 -> [w1736]
                                shift-right: [w1737] -> w1725
                                shift-left: w1727 -> [w1734]
                                n342 = call "Get U64.vi"("Offset"=w1735, "JSON"=w1736) -> ("error out"=w1733:errorcluster, "Number"=w1732:u64)  [unwired: 7 in, 1 out]
                                n343 = Merge Errors(w1734, w1733) -> (w1737:errorcluster)
                                }
                                }
                                frame Error {
                                }
                                }
                                n344 = Merge Errors(w1714, w1724) -> (w1715:errorcluster)
                                }
                              }
                              frame Error {
                              }
                            }
                            n345 = Merge Errors(w1696, w1706) -> (w1697:errorcluster)
                          }
                        }
                        frame Error {
                        }
                      }
                    }
                  }
                }
                frame "Variant".."Waveform", "LabVIEW Class Instance".. {
                  # "Includes Sets and Maps (which follow \"LabVIEW Class Instance\")"
                  n346 = case shown="2" w1746 {
                    tunnel: [w1752 w1763 w1785 w1833] -> w1751
                    tunnel: w1750 -> [w1752 w1758 w1784 w1832]
                    tunnel: w1749 -> [_ w1762 w1789 w1837]
                    tunnel: [w1753 w1760 w1787 w1835] -> w1748
                    tunnel: w1744 -> [_ w1759 w1786 w1834]
                    tunnel: w1747 -> [_ w1755 w1782 w1830]
                    tunnel: w1745 -> [w1753 w1756 _ _]
                    tunnel: w1743 -> [_ _ _ _]
                    tunnel: w1742 -> [_ w1754 w1781 w1829]
                    frame 0, Default {
                    }
                    frame 1 {
                      n347 = call "Get Array Elements (by Offset).vi"("error in (no error)"=w1758, "Offset"=w1759, "JSON"=w1755) -> ("error out"=w1757:errorcluster, "Element Offsets"=w1761:i32[])  [unwired: 5 in, 2 out]
                      n348 = case shown="No Error" w1757 {
                        selector: w1757 -> [w1765 w1779]
                        tunnel: [w1770 w1779] -> w1763
                        tunnel: w1762 -> [w1769 _]
                        tunnel: w1761 -> [w1768 _]
                        tunnel: [w1767 w1780] -> w1760
                        tunnel: w1754 -> [w1766 _]
                        tunnel: w1756 -> [_ w1780]
                        tunnel: w1755 -> [w1764 _]
                        frame No Error {
                          n349 = for {
                            tunnel: w1769 -> [w1778]
                            tunnel: [w1777] -> w1767 mode=indexing
                            tunnel: w1768 -> [w1775] mode=indexing
                            tunnel: w1766 -> [w1771]
                            tunnel: w1764 -> [w1774]
                            shift-right: [w1773] -> w1770
                            shift-left: w1765 -> [w1772]
                            n350 = call "JSON text to Variant.vi"("LVClass Serializer"=w1771, "Data Type"=w1778, "Offset"=w1775, "JSON"=w1774) -> ("error out"=w1776:errorcluster, "Variant out"=w1777:variant)  [unwired: 6 in]
                            n351 = Merge Errors(w1772, w1776) -> (w1773:errorcluster)
                          }
                        }
                        frame Error {
                        }
                      }
                    }
                    frame 2 {
                      n352 = call "Get Array Elements (by Offset).vi"("error in (no error)"=w1784, "Offset"=w1786, "JSON"=w1782) -> ("error out"=w1783:errorcluster, "Element Offsets"=w1788:i32[])  [unwired: 5 in, 2 out]
                      n353 = case shown="No Error" w1783 {
                        selector: w1783 -> [w1792 w1828]
                        tunnel: w1789 -> [w1796 w1827]
                        tunnel: w1788 -> [w1795 _]
                        tunnel: [w1794 w1827] -> w1787
                        tunnel: [w1790 w1828] -> w1785
                        tunnel: w1781 -> [w1793 _]
                        tunnel: w1782 -> [w1791 _]
                        frame No Error {
                          n354 = for {
                            tunnel: w1796 -> [w1806]
                            tunnel: w1795 -> [w1801] mode=indexing
                            tunnel: [w1805] -> w1794 mode=indexing
                            tunnel: w1793 -> [w1803]
                            tunnel: w1791 -> [w1800]
                            tunnel: w1791 -> [w1799]
                            shift-right: [w1798] -> w1790
                            shift-left: w1792 -> [w1797]
                            n355 = call "Get Array Elements (by Offset).vi"("Offset"=w1801, "JSON"=w1800) -> ("error out"=w1802:errorcluster, "Element Offsets"=w1804:i32[])  [unwired: 6 in, 2 out]
                            n356 = case shown="No Error" w1802 {
                              selector: w1802 -> [w1810 w1826]
                              tunnel: [w1808 w1826] -> w1807
                              tunnel: w1806 -> [w1814 w1824]
                              tunnel: [w1813 w1823] -> w1805
                              tunnel: w1804 -> [w1812 _]
                              tunnel: w1803 -> [w1811 _]
                              tunnel: w1799 -> [w1809 _]
                              frame No Error {
                                n357 = for {
                                tunnel: w1814 -> [w1820]
                                tunnel: [w1822] -> w1813 mode=indexing
                                tunnel: w1812 -> [w1818] mode=indexing
                                tunnel: w1811 -> [w1819]
                                tunnel: w1809 -> [w1817]
                                shift-right: [w1816] -> w1808
                                shift-left: w1810 -> [w1815]
                                n358 = call "JSON text to Variant.vi"("LVClass Serializer"=w1819, "Data Type"=w1820, "Offset"=w1818, "JSON"=w1817) -> ("error out"=w1821:errorcluster, "Variant out"=w1822:variant)  [unwired: 6 in]
                                n359 = Merge Errors(w1815, w1821) -> (w1816:errorcluster)
                                }
                              }
                              frame Error {
                                n360 = Initialize Array(w1824, 0 ("dimension size")) -> (w1823:variant[])
                              }
                            }
                            n361 = Merge Errors(w1797, w1807) -> (w1798:errorcluster)
                          }
                        }
                        frame Error {
                        }
                      }
                    }
                    frame 3 {
                      n362 = call "Get Array Elements (by Offset).vi"("error in (no error)"=w1832, "Offset"=w1834, "JSON"=w1830) -> ("error out"=w1831:errorcluster, "Element Offsets"=w1836:i32[])  [unwired: 5 in, 2 out]
                      n363 = case shown="No Error" w1831 {
                        selector: w1831 -> [w1840 w1897]
                        tunnel: w1837 -> [w1844 w1896]
                        tunnel: w1836 -> [w1843 _]
                        tunnel: [w1842 w1896] -> w1835
                        tunnel: [w1838 w1897] -> w1833
                        tunnel: w1829 -> [w1841 _]
                        tunnel: w1830 -> [w1839 _]
                        frame No Error {
                          n364 = for {
                            tunnel: w1844 -> [w1854]
                            tunnel: w1843 -> [w1849] mode=indexing
                            tunnel: [w1853] -> w1842 mode=indexing
                            tunnel: w1841 -> [w1851]
                            tunnel: w1839 -> [w1848]
                            tunnel: w1839 -> [w1847]
                            shift-right: [w1846] -> w1838
                            shift-left: w1840 -> [w1845]
                            n365 = call "Get Array Elements (by Offset).vi"("Offset"=w1849, "JSON"=w1848) -> ("error out"=w1850:errorcluster, "Element Offsets"=w1852:i32[])  [unwired: 6 in, 2 out]
                            n366 = case shown="No Error" w1850 {
                              selector: w1850 -> [w1856 w1895]
                              tunnel: [w1858 w1895] -> w1855
                              tunnel: w1854 -> [w1862 w1894]
                              tunnel: [w1857 w1892] -> w1853
                              tunnel: w1852 -> [w1861 _]
                              tunnel: w1851 -> [w1859 _]
                              tunnel: w1847 -> [w1860 _]
                              frame No Error {
                                n367 = for {
                                tunnel: w1862 -> [w1872]
                                tunnel: w1861 -> [w1867] mode=indexing
                                tunnel: [w1871] -> w1857 mode=indexing
                                tunnel: w1859 -> [w1869]
                                tunnel: w1860 -> [w1866]
                                tunnel: w1860 -> [w1865]
                                shift-right: [w1864] -> w1858
                                shift-left: w1856 -> [w1863]
                                n368 = call "Get Array Elements (by Offset).vi"("Offset"=w1867, "JSON"=w1866) -> ("error out"=w1868:errorcluster, "Element Offsets"=w1870:i32[])  [unwired: 6 in, 2 out]
                                n369 = case shown="No Error" w1868 {
                                selector: w1868 -> [w1876 w1890]
                                tunnel: [w1874 w1890] -> w1873
                                tunnel: w1872 -> [w1880 w1891]
                                tunnel: [w1879 w1889] -> w1871
                                tunnel: w1870 -> [w1878 _]
                                tunnel: w1869 -> [w1877 _]
                                tunnel: w1865 -> [w1875 _]
                                frame No Error {
                                n370 = for {
                                tunnel: w1880 -> [w1886]
                                tunnel: [w1888] -> w1879 mode=indexing
                                tunnel: w1878 -> [w1884] mode=indexing
                                tunnel: w1877 -> [w1885]
                                tunnel: w1875 -> [w1883]
                                shift-right: [w1882] -> w1874
                                shift-left: w1876 -> [w1881]
                                n371 = call "JSON text to Variant.vi"("LVClass Serializer"=w1885, "Data Type"=w1886, "Offset"=w1884, "JSON"=w1883) -> ("error out"=w1887:errorcluster, "Variant out"=w1888:variant)  [unwired: 6 in]
                                n372 = Merge Errors(w1881, w1887) -> (w1882:errorcluster)
                                }
                                }
                                frame Error {
                                n373 = Build Array(w1891) -> (w1889:variant[])
                                }
                                }
                                n374 = Merge Errors(w1863, w1873) -> (w1864:errorcluster)
                                }
                              }
                              frame Error {
                                w1893 = 0 ("dimension size")
                                n375 = Initialize Array(w1894, w1893, w1893) -> (w1892:variant[][])
                              }
                            }
                            n376 = Merge Errors(w1845, w1855) -> (w1846:errorcluster)
                          }
                        }
                        frame Error {
                        }
                      }
                    }
                  }
                }
                frame "Cluster" {
                  n377 = case shown="2" w1902 {
                    tunnel: [w1908 w1920 w1961] -> w1907
                    tunnel: w1906 -> [w1908 w1915 w1960]
                    tunnel: w1905 -> [_ w1919 w1965]
                    tunnel: [w1909 w1917 w1963] -> w1904
                    tunnel: w1900 -> [_ w1916 w1962]
                    tunnel: w1903 -> [_ w1912 w1958]
                    tunnel: w1901 -> [w1909 w1913 _]
                    tunnel: w1899 -> [_ w1910 _]
                    tunnel: w1898 -> [_ w1911 w1957]
                    frame 0, Default {
                    }
                    frame 1 {
                      n378 = call "Get Array Elements (by Offset).vi"("error in (no error)"=w1915, "Offset"=w1916, "JSON"=w1912) -> ("error out"=w1914:errorcluster, "Element Offsets"=w1918:i32[])  [unwired: 5 in, 2 out]
                      n379 = case shown="No Error" w1914 {
                        selector: w1914 -> [w1923 w1955]
                        tunnel: [w1928 w1955] -> w1920
                        tunnel: w1919 -> [w1927 _]
                        tunnel: w1918 -> [w1926 _]
                        tunnel: [w1925 w1956] -> w1917
                        tunnel: w1911 -> [w1924 _]
                        tunnel: w1913 -> [_ w1956]
                        tunnel: w1912 -> [w1922 _]
                        tunnel: w1910 -> [w1921 _]
                        frame No Error {
                          n380 = case shown="\"Cluster\"" w1921 {
                            tunnel: [w1933 w1946] -> w1928
                            tunnel: w1927 -> [w1932 w1945]
                            tunnel: w1926 -> [w1930 w1944]
                            tunnel: [w1934 w1943] -> w1925
                            tunnel: w1924 -> [w1929 w1942]
                            tunnel: w1923 -> [w1931 w1941]
                            tunnel: w1922 -> [w1935 w1940]
                            frame "Cluster" {
                              n381 = call "JSON to Cluster Preparation.vi"("error in (no error)"=w1931, "Cluster"=w1932) -> ("error out"=w1939:errorcluster, "Element Info"=w1936:T4, "Elements"=w1938:variant[], "ELement Names (as JSON)"=w1937:string[])  [unwired: 6 in]
                              n382 = call "JSON to Array of Cluster.vi"("JSON"=w1935, "JSONtext LVClass Serializer in"=w1929, "Item Offset"=w1930, "error in (no error)"=w1939, "Element Info"=w1936, "Elements"=w1938, "ELement Names"=w1937) -> ("error out"=w1933:errorcluster, "Cluster of Variants"=w1934:variant[])  [unwired: 3 in]
                            }
                            frame Default {
                              n383 = for {
                                tunnel: w1945 -> [w1954]
                                tunnel: [w1953] -> w1943 mode=indexing
                                tunnel: w1944 -> [w1951] mode=indexing
                                tunnel: w1942 -> [w1947]
                                tunnel: w1940 -> [w1950]
                                shift-right: [w1949] -> w1946
                                shift-left: w1941 -> [w1948]
                                n384 = call "JSON text to Variant.vi"("LVClass Serializer"=w1947, "Data Type"=w1954, "Offset"=w1951, "JSON"=w1950) -> ("error out"=w1952:errorcluster, "Variant out"=w1953:variant)  [unwired: 6 in]
                                n385 = Merge Errors(w1948, w1952) -> (w1949:errorcluster)
                              }
                            }
                          }
                        }
                        frame Error {
                        }
                      }
                    }
                    frame 2 {
                      n386 = call "Get Array Elements (by Offset).vi"("error in (no error)"=w1960, "Offset"=w1962, "JSON"=w1958) -> ("error out"=w1959:errorcluster, "Element Offsets"=w1964:i32[])  [unwired: 5 in, 2 out]
                      n387 = case shown="No Error" w1959 {
                        selector: w1959 -> [w1969 w2052]
                        tunnel: w1965 -> [w1973 w2051]
                        tunnel: w1964 -> [w1972 _]
                        tunnel: [w1971 w2051] -> w1963
                        tunnel: [w1967 w2052] -> w1961
                        tunnel: w1957 -> [w1970 _]
                        tunnel: w1958 -> [w1968 _]
                        tunnel: w1957 -> [w1966 _]
                        frame No Error {
                          n388 = disable-structure shown="Enabled" {
                            disable-tunnel: w1973 -> [w1980 w2014]
                            disable-tunnel: w1972 -> [w1979 w2022]
                            disable-tunnel: [w1978 w2021] -> w1971
                            disable-tunnel: w1970 -> [w1977 w2020]
                            disable-tunnel: w1969 -> [w1976 w2017]
                            disable-tunnel: w1968 -> [w1975 w2019]
                            disable-tunnel: [w1974 w2018] -> w1967
                            disable-tunnel: w1966 -> [_ w2011]
                            frame Disabled {
                              n389 = for {
                                tunnel: w1980 -> [w1990]
                                tunnel: w1979 -> [w1985] mode=indexing
                                tunnel: [w1989] -> w1978 mode=indexing
                                tunnel: w1977 -> [w1987]
                                tunnel: w1975 -> [w1984]
                                tunnel: w1975 -> [w1983]
                                shift-right: [w1982] -> w1974
                                shift-left: w1976 -> [w1981]
                                n390 = call "Get Array Elements (by Offset).vi"("Offset"=w1985, "JSON"=w1984) -> ("error out"=w1986:errorcluster, "Element Offsets"=w1988:i32[])  [unwired: 6 in, 2 out]
                                n391 = case shown="No Error" w1986 {
                                selector: w1986 -> [w1994 w2010]
                                tunnel: [w1992 w2010] -> w1991
                                tunnel: w1990 -> [w1998 w2008]
                                tunnel: [w1997 w2007] -> w1989
                                tunnel: w1988 -> [w1996 _]
                                tunnel: w1987 -> [w1995 _]
                                tunnel: w1983 -> [w1993 _]
                                frame No Error {
                                n392 = for {
                                tunnel: w1998 -> [w2004]
                                tunnel: [w2006] -> w1997 mode=indexing
                                tunnel: w1996 -> [w2002] mode=indexing
                                tunnel: w1995 -> [w2003]
                                tunnel: w1993 -> [w2001]
                                shift-right: [w2000] -> w1992
                                shift-left: w1994 -> [w1999]
                                n393 = call "JSON text to Variant.vi"("LVClass Serializer"=w2003, "Data Type"=w2004, "Offset"=w2002, "JSON"=w2001) -> ("error out"=w2005:errorcluster, "Variant out"=w2006:variant)  [unwired: 6 in]
                                n394 = Merge Errors(w1999, w2005) -> (w2000:errorcluster)
                                }
                                }
                                frame Error {
                                n395 = Initialize Array(w2008, 0 ("dimension size")) -> (w2007:variant[])
                                }
                                }
                                n396 = Merge Errors(w1981, w1991) -> (w1982:errorcluster)
                              }
                            }
                            frame Enabled {
                              n397 = call "JSON to Cluster Preparation.vi"("error in (no error)"=w2017, "Cluster"=w2014) -> ("error out"=w2015:errorcluster, "Element Info"=w2012:T4, "Elements"=w2013:variant[], "ELement Names (as JSON)"=w2016:string[])  [unwired: 6 in]
                              n398 = for {
                                tunnel: w2016 -> [w2036]
                                tunnel: w2022 -> [w2031] mode=indexing
                                tunnel: [w2035] -> w2021 mode=indexing
                                tunnel: w2020 -> [w2033]
                                tunnel: w2019 -> [w2030]
                                tunnel: w2019 -> [w2029]
                                shift-right: [w2028] -> w2018
                                shift-left: w2015 -> [w2027]
                                tunnel: w2014 -> [w2026]
                                tunnel: w2013 -> [w2025]
                                tunnel: w2012 -> [w2024]
                                tunnel: w2011 -> [w2023]
                                n399 = call "Get Array Elements (by Offset).vi"("Offset"=w2031, "JSON"=w2030) -> ("error out"=w2032:errorcluster, "Element Offsets"=w2034:i32[])  [unwired: 6 in, 2 out]
                                n400 = case shown="No Error" w2032 {
                                selector: w2032 -> [w2043 w2050]
                                tunnel: [w2044 w2050] -> w2037
                                tunnel: w2036 -> [w2046 _]
                                tunnel: [w2045 w2048] -> w2035
                                tunnel: w2034 -> [w2039 _]
                                tunnel: w2033 -> [_ _]
                                tunnel: w2029 -> [w2038 _]
                                tunnel: w2026 -> [_ w2047]
                                tunnel: w2025 -> [w2042 _]
                                tunnel: w2024 -> [w2041 _]
                                tunnel: w2023 -> [w2040 _]
                                frame No Error {
                                n401 = call "JSON to Array of Cluster.vi"("JSON"=w2038, "JSONtext LVClass Serializer in"=w2040, "Item Offset"=w2039, "error in (no error)"=w2043, "Element Info"=w2041, "Elements"=w2042, "ELement Names"=w2046) -> ("error out"=w2044:errorcluster, "Cluster of Variants"=w2045:variant[])  [unwired: 3 in]
                                }
                                frame Error {
                                n402 = Initialize Array(w2047, 0 ("dimension size")) -> (w2048:variant[])
                                }
                                }
                                n403 = Merge Errors(w2027, w2037) -> (w2028:errorcluster)
                              }
                            }
                          }
                        }
                        frame Error {
                        }
                      }
                    }
                  }
                }
                frame "String" {
                  n404 = call "JSON Tags on Array.vi"("Array Name"=w2056, "Element Name"=w2054) -> ("Tag"=w2053:T3)  [unwired: 9 in]
                  n405 = case shown="\"No Tag\", \"<JOBJ>\"" w2053 {
                    tunnel: w2062 -> [w2069 w2107 w2147]
                    tunnel: w2061 -> [w2068 w2106 w2146]
                    tunnel: [w2067 w2105 w2145] -> w2060
                    tunnel: [w2066 w2104 w2144] -> w2059
                    tunnel: w2058 -> [w2065 w2103 w2143]
                    tunnel: w2057 -> [w2064 w2102 w2142]
                    tunnel: w2055 -> [w2063 w2101 w2141]
                    frame "No Tag", "<JOBJ>" {
                      # "#ds issue #2 Can't use LV primative\nbecause it mishandles zero bytes."
                      n406 = case shown="1" w2065 {
                        tunnel: w2069 -> [_ w2076 w2086]
                        tunnel: w2068 -> [w2070 w2073 w2087]
                        tunnel: [w2070 w2074 w2088] -> w2067
                        tunnel: [w2071 w2075 w2089] -> w2066
                        tunnel: w2064 -> [w2071 _ _]
                        tunnel: w2063 -> [_ w2072 w2085]
                        frame 0, Default {
                        }
                        frame 1 {
                          n407 = call "Get Array Elements.vi"("error in (no error)"=w2073, "Offset"=w2072, "JSON"=w2076) -> ("error out"=w2078:errorcluster, "<JSON>"=w2077:string[])  [unwired: 6 in, 1 out]
                          n408 = for {
                            tunnel: w2077 -> [w2082] mode=indexing
                            tunnel: [w2081] -> w2075 mode=indexing
                            shift-right: [w2080] -> w2074
                            shift-left: w2078 -> [w2079]
                            n409 = call "Strip Quotes and Unescape.vi"("error in (no error)"=w2079, "String"=w2082) -> ("error out"=w2080:errorcluster, "result string"=w2081:string)  [unwired: 8 in]
                          }
                        }
                        frame 2 {
                          n410 = call "Get Array Elements (by Offset).vi"("error in (no error)"=w2087, "Offset"=w2085, "JSON"=w2086) -> ("error out"=w2084:errorcluster, "Element Offsets"=w2083:i32[])  [unwired: 5 in, 2 out]
                          n411 = for {
                            tunnel: w2083 -> [w2091] mode=indexing
                            tunnel: [w2094] -> w2089 mode=indexing
                            shift-right: [w2093] -> w2088
                            shift-left: w2084 -> [w2096]
                            tunnel: w2086 -> [w2090]
                            n412 = call "Get Array Elements.vi"("error in (no error)"=w2096, "Offset"=w2091, "JSON"=w2090) -> ("error out"=w2092:errorcluster, "<JSON>"=w2095:string[])  [unwired: 6 in, 1 out]
                            n413 = for {
                              tunnel: w2095 -> [w2100] mode=indexing
                              tunnel: [w2099] -> w2094 mode=indexing
                              shift-right: [w2098] -> w2093
                              shift-left: w2092 -> [w2097]
                              n414 = call "Strip Quotes and Unescape.vi"("error in (no error)"=w2097, "String"=w2100) -> ("error out"=w2098:errorcluster, "result string"=w2099:string)  [unwired: 8 in]
                            }
                          }
                        }
                      }
                    }
                    frame "<UTF8>" {
                      # "#ds issue #2 Can't use LV primative\nbecause it mishandles zero bytes."
                      n415 = case shown="1" w2103 {
                        tunnel: w2107 -> [_ w2114 w2125]
                        tunnel: w2106 -> [w2108 w2111 w2126]
                        tunnel: [w2108 w2112 w2127] -> w2105
                        tunnel: [w2109 w2113 w2128] -> w2104
                        tunnel: w2102 -> [w2109 _ _]
                        tunnel: w2101 -> [_ w2110 w2124]
                        frame 0, Default {
                        }
                        frame 1 {
                          n416 = call "Get Array Elements.vi"("error in (no error)"=w2111, "Offset"=w2110, "JSON"=w2114) -> ("error out"=w2116:errorcluster, "<JSON>"=w2115:string[])  [unwired: 6 in, 1 out]
                          n417 = for {
                            tunnel: w2115 -> [w2121] mode=indexing
                            tunnel: [w2120] -> w2113 mode=indexing
                            shift-right: [w2119] -> w2112
                            shift-left: w2116 -> [w2118]
                            n418 = call "Strip Quotes and Unescape.vi"("error in (no error)"=w2118, "To System Encoding (T)"=FALSE, "String"=w2121) -> ("error out"=w2119:errorcluster, "result string"=w2120:string)  [unwired: 7 in]
                          }
                        }
                        frame 2 {
                          n419 = call "Get Array Elements (by Offset).vi"("error in (no error)"=w2126, "Offset"=w2124, "JSON"=w2125) -> ("error out"=w2123:errorcluster, "Element Offsets"=w2122:i32[])  [unwired: 5 in, 2 out]
                          n420 = for {
                            tunnel: w2122 -> [w2130] mode=indexing
                            tunnel: [w2133] -> w2128 mode=indexing
                            shift-right: [w2132] -> w2127
                            shift-left: w2123 -> [w2135]
                            tunnel: w2125 -> [w2129]
                            n421 = call "Get Array Elements.vi"("error in (no error)"=w2135, "Offset"=w2130, "JSON"=w2129) -> ("error out"=w2131:errorcluster, "<JSON>"=w2134:string[])  [unwired: 6 in, 1 out]
                            n422 = for {
                              tunnel: w2134 -> [w2140] mode=indexing
                              tunnel: [w2139] -> w2133 mode=indexing
                              shift-right: [w2138] -> w2132
                              shift-left: w2131 -> [w2137]
                              n423 = call "Strip Quotes and Unescape.vi"("error in (no error)"=w2137, "To System Encoding (T)"=FALSE, "String"=w2140) -> ("error out"=w2138:errorcluster, "result string"=w2139:string)  [unwired: 7 in]
                            }
                          }
                        }
                      }
                    }
                    frame "<JSON>" {
                      # "JSON text"
                      n424 = case shown="2" w2143 {
                        tunnel: w2147 -> [_ w2154 w2158]
                        tunnel: w2146 -> [w2148 w2153 w2159]
                        tunnel: [w2148 w2152 w2160] -> w2145
                        tunnel: [w2149 w2151 w2161] -> w2144
                        tunnel: w2142 -> [w2149 _ _]
                        tunnel: w2141 -> [_ w2150 w2157]
                        frame 0, Default {
                        }
                        frame 1 {
                          n425 = call "Get Array Elements.vi"("error in (no error)"=w2153, "Offset"=w2150, "JSON"=w2154) -> ("error out"=w2152:errorcluster, "<JSON>"=w2151:string[])  [unwired: 6 in, 1 out]
                        }
                        frame 2 {
                          # "#98"
                          n426 = call "Get Array Elements (by Offset).vi"("error in (no error)"=w2159, "Offset"=w2157, "JSON"=w2158) -> ("error out"=w2156:errorcluster, "Element Offsets"=w2155:i32[])  [unwired: 5 in, 2 out]
                          n427 = for {
                            tunnel: w2155 -> [w2163] mode=indexing
                            tunnel: [w2164] -> w2161 mode=indexing
                            shift-right: [w2165] -> w2160
                            shift-left: w2156 -> [w2166]
                            tunnel: w2158 -> [w2162]
                            n428 = call "Get Array Elements.vi"("error in (no error)"=w2166, "Offset"=w2163, "JSON"=w2162) -> ("error out"=w2165:errorcluster, "<JSON>"=w2164:string[])  [unwired: 6 in, 1 out]
                          }
                        }
                      }
                    }
                  }
                }
              }
            }
          }
        }
        frame Error {
        }
      }
    }
    frame "Waveform" {
      # "Attributes not supported"
      n429 = Variant To Data(error in=w2186, type=waveform(dbl) {"t0"=timestamp(0 s since 1904-01-01), "dt"=1.0, "Y"=[]} ("waveform"), Variant=w2187) -> (data=w2169:waveform(dbl), error out=w2179:errorcluster)
      n430 = Unbundle By Name(w2169) -> ("t0"=w2184:timestamp, "dt"=w2183:dbl, "Y"=w2182:dbl[])  [unwired: 1 out]
      n431 = Bundle("t0"=w2184, "dt"=w2183, "Y"=w2182) -> (w2176:cluster{"t0":timestamp, "dt":dbl, "Y":dbl[]})  [unwired: 1 in]
      n432 = call "JSON text to Variant.vi"("LVClass Serializer"=w2170, "error in (no error)"=w2179, "Data Type"=w2176, "Offset"=w2180, "JSON"=w2181) -> ("error out"=w2178:errorcluster, "Variant out"=w2177:variant)  [unwired: 5 in]
      n433 = Variant To Data(type=w2176, Variant=w2177) -> (data=w2175:cluster{"t0":timestamp, "dt":dbl, "Y":dbl[]})  [unwired: 1 in, 1 out]
      n434 = Unbundle By Name(w2175) -> ("t0"=w2174:timestamp, "dt"=w2173:dbl, "Y"=w2172:dbl[])
      n435 = Bundle By Name("t0"=w2174, "dt"=w2173, "Y"=w2172) -> (w2171:waveform(dbl))  [unwired: 1 in]
    }
    frame "Cluster" {
      n436 = case "JSON type" shown="\"Object\", \"Array\"" w2188 {
        tunnel: w2195 -> [w2200 w2215]
        tunnel: w2194 -> [w2199 w2214]
        tunnel: [w2200 w2210] -> w2191
        tunnel: [w2201 w2213] -> w2193
        tunnel: w2192 -> [w2198 w2212]
        tunnel: w2189 -> [w2197 w2211]
        tunnel: w2190 -> [_ w2209]
        frame Default {
          # "Issue #65"
          n437 = call "JSON type.vi"("Offset"=w2197, "JSON"=w2198) -> ("JSON Value Type"=w2196:T5)  [unwired: 8 in, 1 out]
          n438 = Format Into String(w2196) -> (resulting string=w2202:string)  [unwired: 3 in, 1 out]
          n439 = call "Format Error.vi"("error code (402842)"=402844, "error in (no error)"=w2199, "message part 2"=w2202, "error message"="Cannot Get as a Cluster: " ("format string")) -> ("error out"=w2201:errorcluster)  [unwired: 7 in]
        }
        frame "Object", "Array" {
          n440 = call "JSON to Cluster Preparation.vi"("error in (no error)"=w2214, "Cluster"=w2215) -> ("error out"=w2208:errorcluster, "Element Info"=w2205:T4, "Elements"=w2207:variant[], "ELement Names (as JSON)"=w2206:string[])  [unwired: 6 in]
          n441 = call "JSON to Cluster.vi"("JSON"=w2212, "JSONtext LVClass Serializer in"=w2209, "Item Offset"=w2211, "error in (no error)"=w2208, "Element Info"=w2205, "Elements"=w2207, "ELement Names (as JSON)"=w2206) -> ("error out"=w2213:errorcluster, "Cluster of Variants"=w2210:variant)  [unwired: 3 in]
        }
      }
    }
    frame "Variant", "LV Variant" {
      # "Unwrap and rewrap"
      n442 = Variant To Data(error in=w2225, type=variant, Variant=w2226) -> (data=w2217:variant, error out=w2222:errorcluster)
      n443 = call "JSON text to Variant.vi"("LVClass Serializer"=w2216, "error in (no error)"=w2222, "Data Type"=w2217, "Offset"=w2220, "JSON"=w2221) -> ("error out"=w2218:errorcluster, "Variant out"=w2219:variant)  [unwired: 5 in]
      n444 = To Variant(anything=w2219) -> (Variant=w2223:variant)
    }
    frame "LabVIEW Class Instance" {
      n445 = Variant To Data(error in=w2235, type=refnum<class> refnum ("LabVIEW Object"), Variant=w2237) -> (data=w2233:refnum<class>, error out=w2236:errorcluster)
      n446 = Not Equal?(x=w2229, y=refnum<class "JSONtext LVClass Serializer.lvclass"> refnum) -> (x != y?=w2227:bool)
      n447 = case shown="False" w2227 {
        tunnel: w2229 -> [_ w2251]
        tunnel: w2238 -> [w2244 w2250]
        tunnel: w2236 -> [w2240 w2249]
        tunnel: w2233 -> [w2239 w2248]
        tunnel: [w2242 w2247] -> w2232
        tunnel: [w2241 w2246] -> w2231
        tunnel: w2230 -> [w2243 w2245]
        frame False {
          n448 = call "JSON to LVObject.vi"("error in (no error)"=w2240, "JSON"=w2244, "Offset of first non-whitespace"=w2243, "LabVIEW Object in"=w2239) -> ("error out"=w2241:errorcluster, "LabVIEW Object out"=w2242:refnum<class>)  [unwired: 6 in]
        }
        frame True {
          # "Issue #56 Way of providing alternate format\nof LVObjects"
          n449 = call-dynamic "JSON to LVObject.vi"("JSONtext LVClass Serializer in"=w2251, "error in (no error)"=w2249, "Object Type"=w2248, "Offset"=w2245, "JSON"=w2250) -> ("error out"=w2246:errorcluster, "Object"=w2247:refnum<class>)  [unwired: 5 in]
        }
      }
    }
    frame "Fixed Point".. {
      n450 = Type Cast(type=u8 0, x=w2257) -> (*(type *) &x=w2260:u8)
      n451 = case shown="47" w2260 {
        tunnel: w2259 -> [w2263 w2270 w2273 w2280]
        tunnel: w2258 -> [_ w2269 w2275 w2282]
        tunnel: w2257 -> [_ w2268 _ _]
        tunnel: w2256 -> [_ w2267 w2271 w2279]
        tunnel: [w2263 w2266 w2272 w2278] -> w2255
        tunnel: w2254 -> [w2262 w2265 w2277 w2284]
        tunnel: [w2262 w2264 w2276 w2283] -> w2253
        tunnel: w2252 -> [_ _ w2274 w2281]
        frame 0, Default {
        }
        frame 45 {
          # "Fixed Point"
          n452 = call "Scalar JSON text to Variant (not inlined).vi"("Type"=w2268, "error in (no error)"=w2265, "Variant (Data Type)"=w2270, "Offset (no whitespace)"=w2267, "JSON"=w2269) -> ("error out"=w2264:errorcluster, "Variant out"=w2266:variant)  [unwired: 5 in]
        }
        frame 46 {
          # "46 == Set in LabVIEW 2019 and later\nIssue #74"
          n453 = call "JSON To Set.vi"("LVClass Serializer"=w2274, "error in (no error)"=w2277, "Set Type"=w2273, "Offset"=w2271, "<JSON>"=w2275) -> ("error out"=w2276:errorcluster, "Set"=w2272:variant)  [unwired: 5 in]
        }
        frame 47 {
          # "47 == Map in LabVIEW 2019 and later\nIssue #74"
          n454 = call "JSON to Map.vi"("LVClass Serializer"=w2281, "error in (no error)"=w2284, "Map Type in"=w2280, "Offset"=w2279, "<JSON>"=w2282) -> ("error out"=w2283:errorcluster, "Map"=w2278:variant)  [unwired: 5 in]
        }
      }
    }
  }
  "Variant out" <- w7
  "error out" <- w9
